vi "Drive Controller.vi"(8 "error in":errorcluster) -> ()   [LabVIEW 2023]
doc: "This VI executes continuously carrying out the current operation and responding to updates or new operation requests. It will often contain the timing or control code that is difficult to place directly in TeleOp. This VI generally opens all sensors and motors and isolates the rest of the robot code from knowing implementation details of how the operations are carried out."
uses:
  Drive Operations.ctl
  bordeaux-pathinator/Bordeaux/Types/Segment Type.ctl
  bordeaux-pathinator/Bordeaux/Types/Limits.ctl
  Drive Setpoints.ctl
  swerve/Type Definitions/Data/Robot Velocities.ctl
  <vilib>/Rock Robotics/WPI/ThirdParty/REV Robotics/REVLib/Typedef/Spark MAX Control Type.ctl
  <vilib>/Rock Robotics/WPI/DriverStation/WPI_DriverStationRobotMode2.ctl
  e7fadf63-5109-474c-80f5-604bef1b4eb3.vi
  80b923c8-6b82-42f9-a8cd-acddf0fa8107.vi
  Framework/Robot Global Data.vi
  <vilib>/Rock Robotics/WPI/ThirdParty/Phoenix-LabVIEW/Pigeon IMU/CTRE_PigeonIMU_GetYPR.vi
  <vilib>/Rock Robotics/Network Tables/NT Write Numeric Array.vi
  <vilib>/Rock Robotics/Network Tables/NT Write String.vi
  <vilib>/Rock Robotics/Network Tables/NT Read Numeric Array.vi
  <vilib>/Rock Robotics/Network Tables/NT Read Number.vi
  <vilib>/Platform/TimedLoop/XDataNode/XDataNode.xnode
  <vilib>/Platform/TimedLoop/XDataNode/nitl_modes.ctl
  <vilib>/Platform/TimedLoop/XDataNode/XDNodeRunTimeDep.lvlib
  <vilib>/Platform/TimedLoop/XDataNode/wakeup.ctl
  <vilib>/Platform/TimedLoop/XDataNode/timing_clust.ctl
  <vilib>/ptbypt/NI_PtbyPt.lvlib
panel:
  out "Error":T1
  in  "Limits":T2={"Velocity (fps)"=10.0, "Accel (fps^2)"=22.0, "Jerk (fps^3)"=4000.0, "StoopidFast (fps)"=10.0} {"StoopidFast (fps)" min=0.0; "Jerk (fps^3)" min=0.0 step=1.0; "Accel (fps^2)" min=0.0; "Velocity (fps)" min=0.0}
  in  "Final Postion":T1={"X setpoint"=13.0, "Y setpoint"=8.0, "Theta"=0.0}
  out "Yaw":dbl=3.92486572265625
  in  "Y Setpoint":dbl=-0.8
  in  "Right PID Setpoint":dbl=0.56
  in  "Left PID Setpoint":dbl=-0.545
  in  "Freeze Align?":bool
  out "VMag Sum":dbl=1.7248000000000006
  out "Enabled VMag":dbl[](graph)=[0.44, 0.88, 1.32, 1.76, 2.2, 2.64, 3.08, 3.52, 3.96, 4.4, 4.840000000000001, 5.280000000000001, 5.7200000000000015, 6.160000000000002, 5.7200000000000015, 5.280000000000001, 4.840000000000001, 4.4, 3.9600000000000004, 3.5200000000000005, 3.0800000000000005, 2.6400000000000006, 2.2000000000000006, 1.7600000000000007, 1.3200000000000007, 1.3200000000000007]
  out "Sum Angle":dbl=-0.25517736196517943
  out "Sum Y":dbl=1.7237185415021776
  out "Sum X":dbl=-0.061040277189923345
  out "Enabled Omega":dbl[](graph)=[-0.0, -0.554733395576477, -0.554733395576477, -0.554733395576477, -0.554733395576477, -0.554733395576477, -0.554733395576477, -0.554733395576477, -0.554733395576477, -0.554733395576477, -0.554733395576477, -0.554733395576477, -0.554733395576477, -0.554733395576477, -0.554733395576477, -0.554733395576477, -0.554733395576477, -0.554733395576477, -0.554733395576477, -0.554733395576477, -0.554733395576477, -0.554733395576477, -0.554733395576477, -0.554733395576477, -0.0, -0.0]
  out "Enabled Y Velocity":dbl[](graph)=[0.4397620571088689, 0.8795184944701074, 1.3192692626162588, 1.7590143120802895, 2.1987535933955944, 2.6384870570959973, 3.0782146537157553, 3.517936333789562, 3.9576520478525503, 4.397361746440296, 4.837065380088821, 5.276762899334593, 5.7164542547145345, 6.1561393967660205, 5.7163758392233, 5.2766181322765675, 4.836866325390256, 4.397120468028349, 3.9573806096543764, 3.5176467997314127, 3.0779190877220737, 2.638197523088511, 2.1984821552924134, 1.7587730337949996, 1.31907977534625, 1.319075836091112]
  out "Enabled X Velocity":dbl[](graph)=[-0.014468349158626874, -0.02910700749021977, -0.04391597335768957, -0.05889524511117701, -0.07404482108804894, -0.0893646996129026, -0.10485487899756332, -0.12051535754108665, -0.13634613352975256, -0.15234720523707615, -0.16851857092379446, -0.1848602288378793, -0.2013721772145311, -0.21805441427617603, -0.2035860131348127, -0.18894731046023522, -0.17413830797893487, -0.1591590074301729, -0.14400941056597527, -0.12868951915114632, -0.1131993349632539, -0.09753885979264178, -0.08170809544241993, -0.06570704372847282, -0.049280282796354616, -0.04938561167522259]
  out "Trajectory Velocity":dbl[](graph)
  out "Trajectory Data Compare":T4(array[cluster])
  out "Trajectory Data Out":T4(array[cluster])=[{"Segment Name"="Linear 0", "Type"=enum."Accel Straight", "Traj Pos Points"=[{"x"=-0.40649778342800347, "y"=-2.496126393436387, "th"=0.25975245237350464}, {"x"=-0.4068270208391716, "y"=-2.4873325545291127, "th"=0.2486577844619751}, {"x"=-0.4074854956615079, "y"=-2.4697448767145644, "th"=0.23756311655044554}, {"x"=-0.40847320789501235, "y"=-2.443363359992742, "th"=0.22646844863891602}, {"x"=-0.40979015753968495, "y"=-2.408188004363646, "th"=0.21537378072738647}, {"x"=-0.4114363445955257, "y"=-2.3642188098272756, "th"=0.20427911281585692}, {"x"=-0.4134117690625346, "y"=-2.311455776383631, "th"=0.1931844449043274}, {"x"=-0.41571643094071165, "y"=-2.2498989040327126, "th"=0.18208977699279785}, {"x"=-0.41835033023005685, "y"=-2.17954819277452, "th"=0.1709951090812683}, {"x"=-0.4213134669305702, "y"=-2.100403642609053, "th"=0.15990044116973876}, {"x"=-0.4246058410422517, "y"=-2.0124652535363126, "th"=0.1488057732582092}, {"x"=-0.42822745256510136, "y"=-1.9157330255562977, "th"=0.13771110534667966}, {"x"=-0.4321783014991192, "y"=-1.8102069586690088, "th"=0.1266164374351501}, {"x"=-0.43645838784430513, "y"=-1.6958870528744459, "th"=0.11552176952362056}, {"x"=-0.4410677116006592, "y"=-1.5727733081726087, "th"=0.10442710161209101}, {"x"=-0.44534779794584517, "y"=-1.4584534023780458, "th"=0.09333243370056146}, {"x"=-0.449298646879863, "y"=-1.352927335490757, "th"=0.08223776578903191}, {"x"=-0.45292025840271266, "y"=-1.256195107510742, "th"=0.07114309787750236}, {"x"=-0.45621263251439415, "y"=-1.1682567184380013, "th"=0.060048429965972816}, {"x"=-0.4591757692149075, "y"=-1.0891121682725347, "th"=0.04895376205444327}, {"x"=-0.4618096685042527, "y"=-1.018761457014342, "th"=0.03785909414291372}, {"x"=-0.4641143303824298, "y"=-0.9572045846634234, "th"=0.02676442623138417}, {"x"=-0.46608975484943865, "y"=-0.904441551219779, "th"=0.01566975831985462}, {"x"=-0.4677359419052794, "y"=-0.8604723566834086, "th"=0.0045750904083251}, {"x"=-0.469052891549952, "y"=-0.8252970010543123, "th"=0.0045750904083251}, {"x"=-0.47004060378345647, "y"=-0.79891548433249, "th"=0.0}], "Traj Vel Points"=[{"V"=0.44, "Omega"=-0.0, "V vector"={"y"=-0.4397620571088689, "x"=-0.014468349158626874}}, {"V"=0.88, "Omega"=-0.554733395576477, "V vector"={"y"=-0.8795184944701074, "x"=-0.02910700749021977}}, {"V"=1.32, "Omega"=-0.554733395576477, "V vector"={"y"=-1.3192692626162588, "x"=-0.04391597335768957}}, {"V"=1.76, "Omega"=-0.554733395576477, "V vector"={"y"=-1.7590143120802895, "x"=-0.05889524511117701}}, {"V"=2.2, "Omega"=-0.554733395576477, "V vector"={"y"=-2.1987535933955944, "x"=-0.07404482108804894}}, {"V"=2.64, "Omega"=-0.554733395576477, "V vector"={"y"=-2.6384870570959973, "x"=-0.0893646996129026}}, {"V"=3.08, "Omega"=-0.554733395576477, "V vector"={"y"=-3.0782146537157553, "x"=-0.10485487899756332}}, {"V"=3.52, "Omega"=-0.554733395576477, "V vector"={"y"=-3.517936333789562, "x"=-0.12051535754108665}}, {"V"=3.96, "Omega"=-0.554733395576477, "V vector"={"y"=-3.9576520478525503, "x"=-0.13634613352975256}}, {"V"=4.4, "Omega"=-0.554733395576477, "V vector"={"y"=-4.397361746440296, "x"=-0.15234720523707615}}, {"V"=4.840000000000001, "Omega"=-0.554733395576477, "V vector"={"y"=-4.837065380088821, "x"=-0.16851857092379446}}, {"V"=5.280000000000001, "Omega"=-0.554733395576477, "V vector"={"y"=-5.276762899334593, "x"=-0.1848602288378793}}, {"V"=5.7200000000000015, "Omega"=-0.554733395576477, "V vector"={"y"=-5.7164542547145345, "x"=-0.2013721772145311}}, {"V"=6.160000000000002, "Omega"=-0.554733395576477, "V vector"={"y"=-6.1561393967660205, "x"=-0.21805441427617603}}, {"V"=5.7200000000000015, "Omega"=-0.554733395576477, "V vector"={"y"=-5.7163758392233, "x"=-0.2035860131348127}}, {"V"=5.280000000000001, "Omega"=-0.554733395576477, "V vector"={"y"=-5.2766181322765675, "x"=-0.18894731046023522}}, {"V"=4.840000000000001, "Omega"=-0.554733395576477, "V vector"={"y"=-4.836866325390256, "x"=-0.17413830797893487}}, {"V"=4.4, "Omega"=-0.554733395576477, "V vector"={"y"=-4.397120468028349, "x"=-0.1591590074301729}}, {"V"=3.9600000000000004, "Omega"=-0.554733395576477, "V vector"={"y"=-3.9573806096543764, "x"=-0.14400941056597527}}, {"V"=3.5200000000000005, "Omega"=-0.554733395576477, "V vector"={"y"=-3.5176467997314127, "x"=-0.12868951915114632}}, {"V"=3.0800000000000005, "Omega"=-0.554733395576477, "V vector"={"y"=-3.0779190877220737, "x"=-0.1131993349632539}}, {"V"=2.6400000000000006, "Omega"=-0.554733395576477, "V vector"={"y"=-2.638197523088511, "x"=-0.09753885979264178}}, {"V"=2.2000000000000006, "Omega"=-0.554733395576477, "V vector"={"y"=-2.1984821552924134, "x"=-0.08170809544241993}}, {"V"=1.7600000000000007, "Omega"=-0.554733395576477, "V vector"={"y"=-1.7587730337949996, "x"=-0.06570704372847282}}, {"V"=1.3200000000000007, "Omega"=-0.0, "V vector"={"y"=-1.31907977534625, "x"=-0.049280282796354616}}, {"V"=1.3200000000000007, "Omega"=-0.0, "V vector"={"y"=-1.319075836091112, "x"=-0.04938561167522259}}], "Accel Index"=14, "Decel Index"=14}, {"Segment Name"="", "Type"=enum."Accel Straight", "Traj Pos Points"=[], "Traj Vel Points"=[], "Accel Index"=0, "Decel Index"=0}]
  in  "PID enabled":bool=TRUE
  out "Trapezoid Profile":dbl[](graph)
  out "Weird Aligning Code?":string
  in  "Go Up?":i32
  in  "Int per ft":dbl=0.75
  in  "PID gains":T5={"proportional gain (Kp)"=1.5, "integral time (Ki)"=0.075, "derivative time (Kd)"=0.0} {"derivative time (Kd)" format="%.3f"; "integral time (Ki)" format="%.3f"; "proportional gain (Kp)" format="%.3f"}
  out "PID Out":dbl=0.10498956284304024
  out "Waveform Chart":cluster{dbl, "Right X Setpoint":dbl}(graph)={-0.574331443611901, "Right X Setpoint"=-0.559167}
  in  "Operation":T6
  in  "Auto PID Constants":T7={"P Gain"=0.09, "I Gain"=0.0, "D Gain"=0.0, "F Gain"=0.08, "I Zone"=0.0, "Min Output"=-1.0, "Max Output"=1.0}
  in  "Immediate PID Constants":T7={"P Gain"=0.09, "I Gain"=0.0, "D Gain"=0.0, "F Gain"=0.08, "I Zone"=0.0, "Min Output"=-1.0, "Max Output"=1.0}
  out "Waveform Chart":cluster{"Numeric":dbl, "Numeric":dbl}(graph)
  in  "Period":i32=26
  in  "Acceleration Max":dbl=3.0
  in  "Velocity Max":dbl=6.0
  in  "Left X Setpoint":dbl=-0.47
  in  "Left Y Setpoint":dbl
  in  "Right Y Setpoint":dbl
  in  "Right X Setpoint":dbl=0.47
  in  "Deadband":T8={"Angle (deg)"=3.0, "X (ft)"=0.1, "Y (ft)"=0.125}
  in  "Drive Controller Diagnostics":T9(tab)
  out "Swerve Visualizer":cluster{dbl[], dbl[]}[](graph)
  out "Pod Comparisons (Diff -> Setpoint - Actual)":T10
  out "(Calibration) Steering Angles":T11={"Left Front"=97.29912567138672, "Left Back"=4.939062595367432, "Right Front"=-174.1834259033203, "Right Back"=-81.83795166015625}
  out "Current\nCmd":string="Started at  16:32:32.148\n: Immediate,  Vx 0.0, Vy -0.0, W -0.000000"
  # "Align Variables"
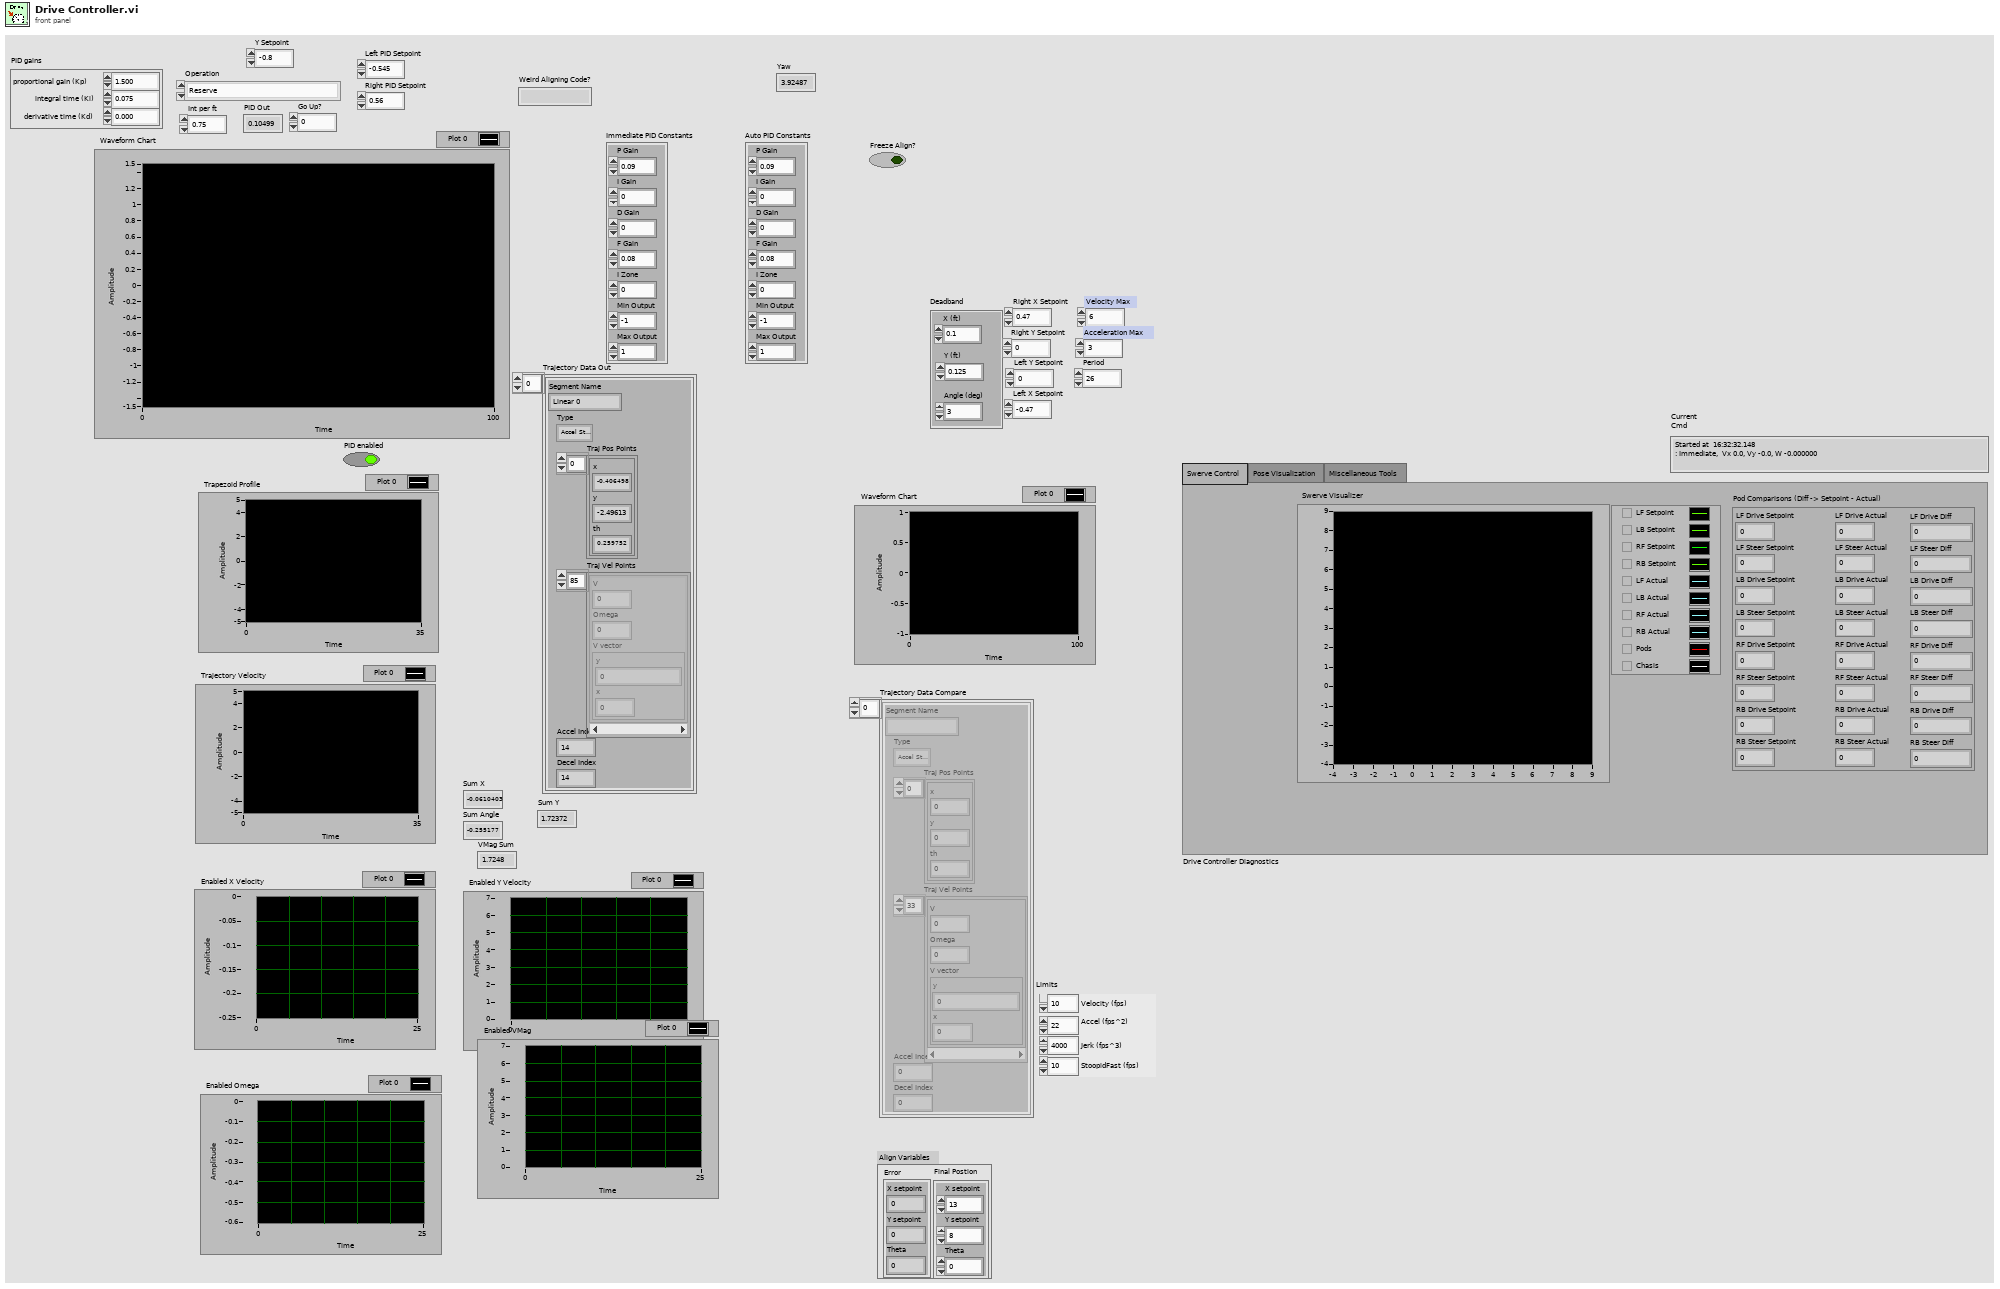
[diagram p1: front panel]
types:
  T1 = cluster{"X setpoint":dbl, "Y setpoint":dbl, "Theta":dbl}
  T2 = typedef "Limits.ctl" = cluster{"Velocity (fps)":dbl, "Accel (fps^2)":dbl, "Jerk (fps^3)":dbl, "StoopidFast (fps)":dbl}
  T3 = typedef "Segment Type.ctl" = enum16{"Accel Straight", "Const Straight", "Blend", "Circle", "Bezier"}
  T4 = cluster{"Segment Name":string, "Type":T3, "Traj Pos Points":cluster{"x":dbl, "y":dbl, "th":dbl}[], "Traj Vel Points":cluster{"V":dbl, "Omega":dbl, "V vector":cluster{"y":dbl, "x":dbl}}[], "Accel Index":i32, "Decel Index":i32}[]
  T5 = cluster{"proportional gain (Kp)":dbl, "integral time (Ki)":dbl, "derivative time (Kd)":dbl}
  T6 = typedef "Drive Operations.ctl" = enum16{"Reserve", "Read Current", "Immediate", "Calibrate", "Reef Align", "Auto", "Old Reef Align"}
  T7 = cluster{"P Gain":dbl, "I Gain":dbl, "D Gain":dbl, "F Gain":dbl, "I Zone":dbl, "Min Output":dbl, "Max Output":dbl}
  T8 = cluster{"Angle (deg)":dbl, "X (ft)":dbl, "Y (ft)":dbl}
  T9 = enum32{"Swerve Control", "Pose Visualization", "Miscellaneous Tools"}
  T10 = cluster{"LF Drive Setpoint":dbl, "LF Steer Setpoint":dbl, "LB Drive Setpoint":dbl, "LB Steer Setpoint":dbl, "RF Drive Setpoint":dbl, "RF Steer Setpoint":dbl, "RB Drive Setpoint":dbl, "RB Steer Setpoint":dbl, "LF Drive Actual":dbl, "LF Steer Actual":dbl, "LB Drive Actual":dbl, "LB Steer Actual":dbl, "RF Drive Actual":dbl, "RF Steer Actual":dbl, "RB Drive Actual":dbl, "RB Steer Actual":dbl, "LF Drive Diff":dbl, "LF Steer Diff":dbl, "LB Drive Diff":dbl, "LB Steer Diff":dbl, "RF Drive Diff":dbl, "RF Steer Diff":dbl, "RB Drive Diff":dbl, "RB Steer Diff":dbl}
  T11 = cluster{"Left Front":dbl, "Left Back":dbl, "Right Front":dbl, "Right Back":dbl}
  T12 = typedef "Drive Setpoints.ctl" = cluster{"Operation":T6, "Robot Velocities":T13, "Auto Data":cluster{"Auto Velocities":T13[], "Auto Positions":cluster{"x":dbl, "y":dbl, "th":dbl}[], "Auto Commands":cluster{dbl, "Command out":cluster{"Name":string, "vi reference":refnum<vi>, i32[], variant[]}}[], "Zero Velocity?":bool[]}, "Left side":bool, "Angle Align":bool, "Tag ID":i32}
  T13 = typedef "Robot Velocities.ctl" = cluster{"X Velocity":dbl, "Y Velocity":dbl, "Rotational \nVelocity":dbl}
  T14 = typedef "(NEO-NEO-ThroughBore-Pigeon2) Swerve.ctl" = cluster{"Drive Motors (NEO)":T15, "Steer Motors (NEO)":T15, "Pigeon2":T21, "Radii (ft)":T23}
  T15 = typedef "(NEO & NEO 550) 4 Motor Set.ctl" = cluster{"Left Front":T16, "Left Back":T16, "Right Front":T16, "Right Back":T16}
  T16 = typedef "WPI_MotorControlDeviceRef.ctl" = cluster{"DeviceStatus":errorcluster, "Type":T17, "PWM":cluster{"PWM Channel":T18, "DeadBand":T19}, "CAN":cluster{"Device Number":u8, "SetOutput VI Ref":variant, "GetOutput VI Ref":variant, "Enable VI Ref":variant, "Disable VI Ref":variant, "Data":variant}, "Invert":bool, "DIO PWM":cluster{"PWM \"Enable\" Channel":T18, "DIOChannel":T20, "PWM Rate":dbl}}
  T17 = typedef "WPI_MotorControlType.ctl" = enum16{"PWM", "CAN", "DIO PWM"}
  T18 = typedef "FPGA_DIOPWMChannel.ctl" = enum8{"PWM 0", "PWM 1", "PWM 2", "PWM 3", "PWM 4", "PWM 5", "PWM 6", "PWM 7", "PWM 8", "PWM 9", "PWM MXP 0", "PWM MXP 1", "PWM MXP 2", "PWM MXP 3", "PWM MXP 4", "PWM MXP 5", "PWM MXP 6", "PWM MXP 7", "PWM MXP 8", "PWM MXP 9", "Invalid"}
  T19 = typedef "WPI_PWMDeadband.ctl" = cluster{"Name":string, "maxPositivePwm":i32, "minPositivePwm":i32, "centerPwm":i32, "maxNegativePwm":i32, "minNegativePwm":i32, "angularRange":u16}
  T20 = typedef "FPGA_DIOChannel.ctl" = enum8{"DIO 0", "DIO 1", "DIO 2", "DIO 3", "DIO 4", "DIO 5", "DIO 6", "DIO 7", "DIO 8", "DIO 9", "DIO MXP 0", "DIO MXP 1", "DIO MXP 2", "DIO MXP 3", "DIO MXP 4", "DIO MXP 5", "DIO MXP 6", "DIO MXP 7", "DIO MXP 8", "DIO MXP 9", "DIO MXP 10", "DIO MXP 11", "DIO MXP 12", "DIO MXP 13", "DIO MXP 14", "DIO MXP 15", "SPI Port CS1", "SPI Port CS2", "SPI Port CS3", "SPI Port MISO", "SPI Port MOSI", "Invalid"}
  T21 = typedef "CTRE_PigeonIMU_DeviceRef.ctl" = cluster{"DeviceStatus":errorcluster, "Device Number":u8, "Type":T22, "Device ID":u32, "Handle":u64, "UsageFrame":u32, "Library Path":path}
  T22 = typedef "CTRE_PigeonIMU_ConnectionType.ctl" = u32
  T23 = typedef "Pod Positions.ctl" = cluster{"Left Front Position":dbl[], "Left Back Position":dbl[], "Right Front Position":dbl[], "Right Back Position":dbl[]}
  T24 = typedef "Command Status Info.ctl" = cluster{"Name":string, "Status":T25, "notifier out":T26}
  T25 = typedef "Completion Status.ctl" = enum16{"Successful", "Aborted", "Incomplete"}
  T26 = typedef "Completion Notifier.ctl" = refnum<notifier>
  T27 = cluster{"SubSystem Data":T12, cluster{"Start Time (ms)":u32, "Iterations":i32}, cluster{"Command Info":T24, "Description":string, "Default Command":T12, "queue out":refnum<queue>, "Subsystem Name":string}}
  T28 = typedef "Spark MAX Control Type.ctl" = enum16{"Percent VBus", "Voltage", "Velocity", "Position", "Smart Motion", "Current", "Smart Velocity", "MAXMotion Position", "MAXMotion Velocity"}
  T29 = typedef "WPI_DriverStationRobotMode2.ctl" = enum16{"Autonomous Disabled", "Autonomous Enabled", "Teleop Disabled", "Teleop Enabled", "Disconnected", "Finish", "Test Disabled", "Test Enabled", "Emergency Stopped"}
  T30 = typedef "XDNodeRunTimeDep.lvlib/timing_clust.ctl" = cluster{"Expected End [f-1]":u64, "Actual End [f-1]":u64, "Finished Late? [f-1]":bool, "Expected End [i-1]":u64, "Actual End [i-1]":u64, "Finished Late? [i-1]":bool, "Expected Start [i]":u64, "Actual Start [i]":u64, "Expected Start [f]":u64, "Actual Start [f]":u64, "Source Name":string, "Structure Name":string, "Period":i64, "Deadline":i64, "Offset":i64, "Start":i64, "Priority":i32, "Timeout":i32, "Mode":T31, "Wakeup Reason":T32, "Error":errorcluster, "Source Type":string, "Secondary Source Type":string, "Global End Time":u64, "Global Start Time":u64, "Frame Duration":u64, "Iteration Duration":u64, "Assigned CPU":i32, "I/O Scan Engine Mode":u32}
  T31 = typedef "XDNodeRunTimeDep.lvlib/nitl_modes.ctl" = enum32{"No Change", "Process missed periods, maintain original phase", "Discard missed periods, maintain original phase", "Process missed periods, ignore original phase", "Discard missed periods, ignore original phase"}
  T32 = typedef "XDNodeRunTimeDep.lvlib/wakeup.ctl" = enum32{"Normal", "Aborted", "Asynchronous wakeup", "Timing source error", "Timed loop error", "Timeout"}
  T33 = cluster{"Auto Velocities":T13[], "Auto Positions":cluster{"x":dbl, "y":dbl, "th":dbl}[], "Auto Commands":cluster{dbl, "Command out":cluster{"Name":string, "vi reference":refnum<vi>, i32[], variant[]}}[], "Zero Velocity?":bool[]}
  T34 = cluster{"Field Centric":bool, "Reef Centric":bool}
  T35 = typedef "Pod Setpoints.ctl" = cluster{"Left Front":cluster{"Velocity":dbl, "Theta":dbl}, "Left Back":cluster{"Velocity":dbl, "Theta":dbl}, "Right Front":cluster{"Velocity":dbl, "Theta":dbl}, "Right Back":cluster{"Velocity":dbl, "Theta":dbl}}
  T36 = cluster{"Left X Setpoint":dbl, "Left Y Setpoint":dbl}
  T37 = cluster{"Right X Setpoint":dbl, "Right Y Setpoint":dbl}
  T38 = cluster{"Segment Name":string, "Type":T3, "Traj Pos Points":cluster{"x":dbl, "y":dbl, "th":dbl}[], "Traj Vel Points":cluster{"V":dbl, "Omega":dbl, "V vector":cluster{"y":dbl, "x":dbl}}[], "Accel Index":i32, "Decel Index":i32}
  T39 = cluster{"V":dbl, "Omega":dbl, "V vector":cluster{"y":dbl, "x":dbl}}[]
  T40 = cluster{"Filtered x":dbl, "Right X Setpoint":dbl}
  T41 = cluster{"Right X Setpoint":dbl, "Y Setpoint":dbl, dbl}
  T42 = cluster{"x setpoint":dbl, "y setpoint":dbl, "th setpoint":dbl}
  T43 = cluster{"SubSystem Data":T12, cluster{"Start Time (ms)":u32, "Iterations":i32}, "Default Command Arguments":cluster{"Command Info":T24, "Description":string, "Default Command":T12, "queue out":refnum<queue>, "Subsystem Name":string}}
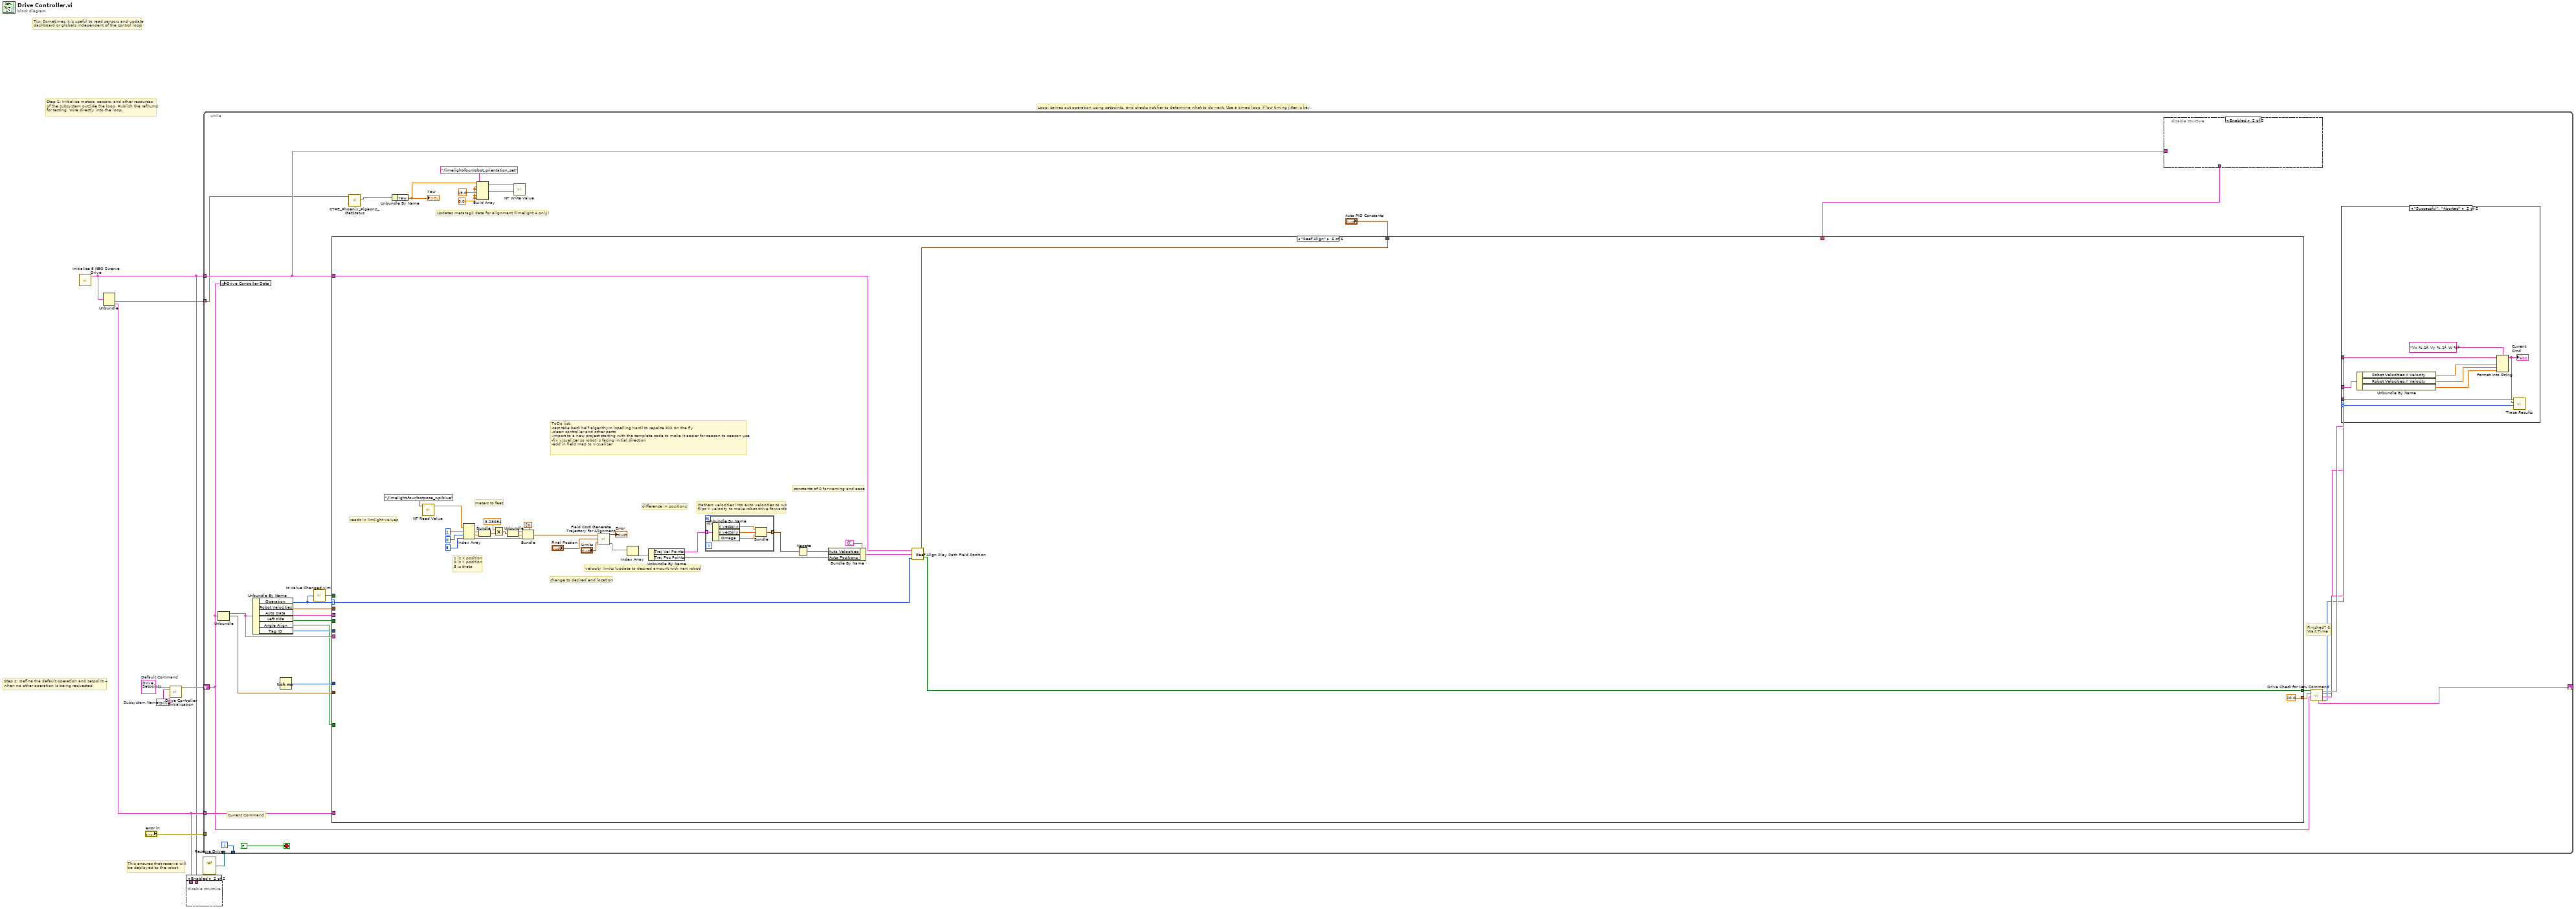
[diagram p0: block diagram]
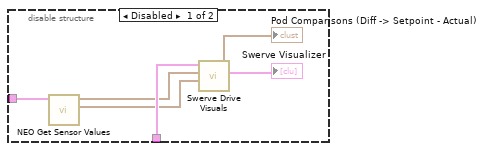
[diagram p2: hidden frame]
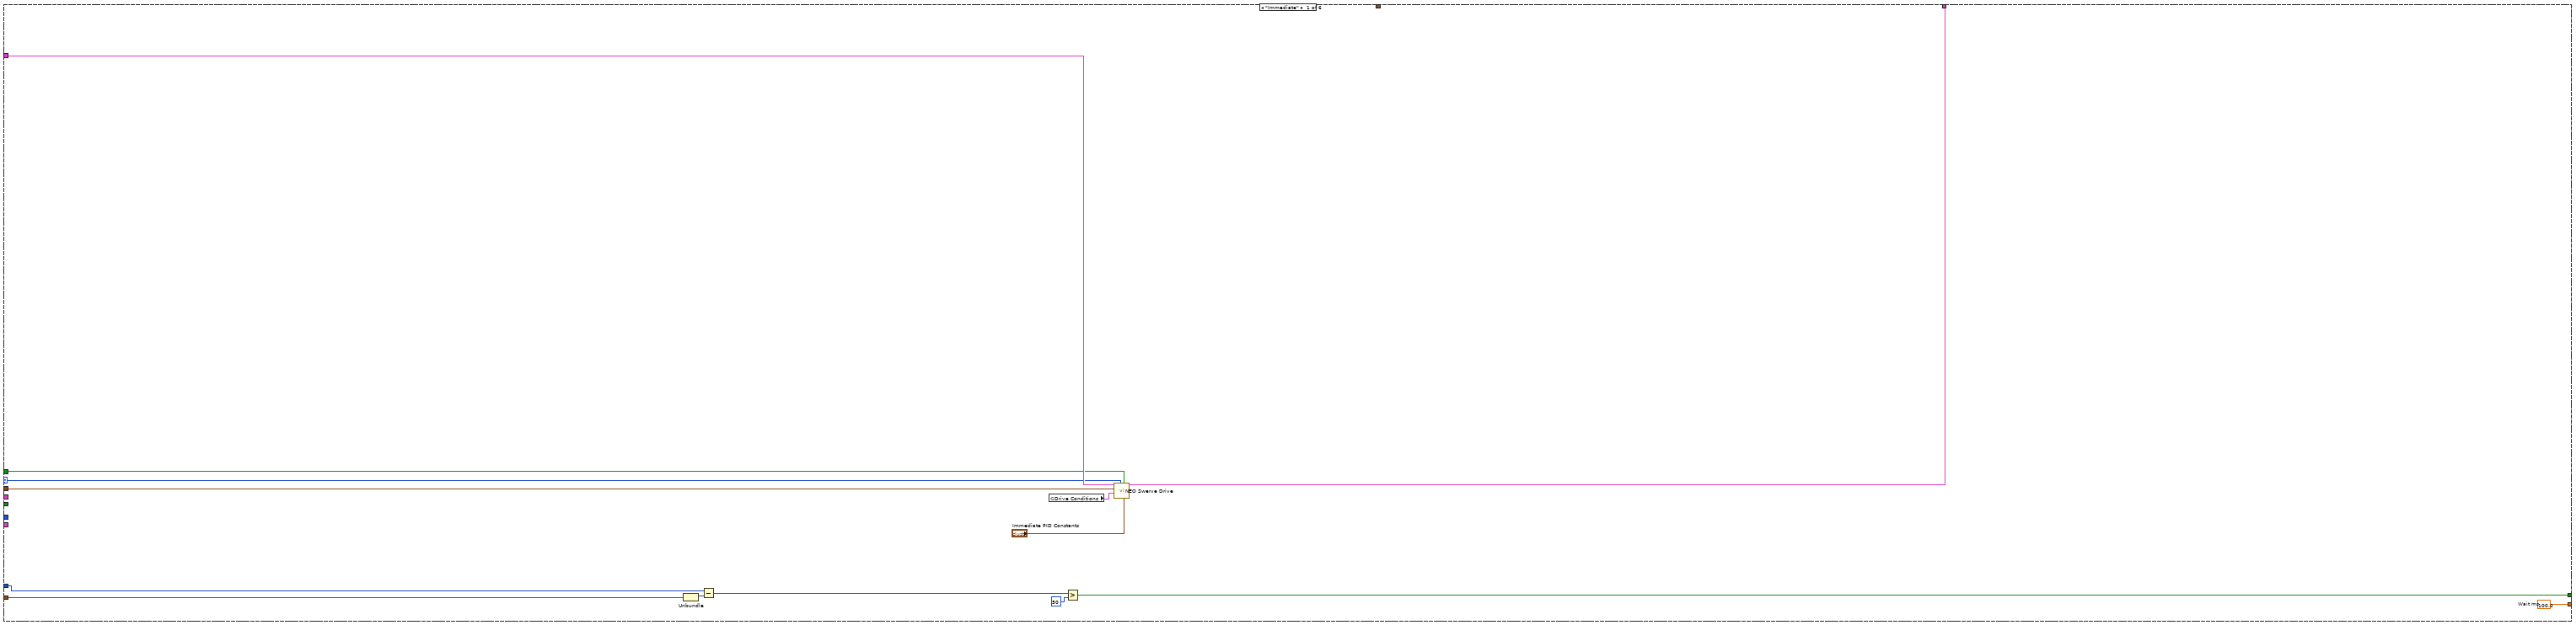
[diagram p3: hidden frame]
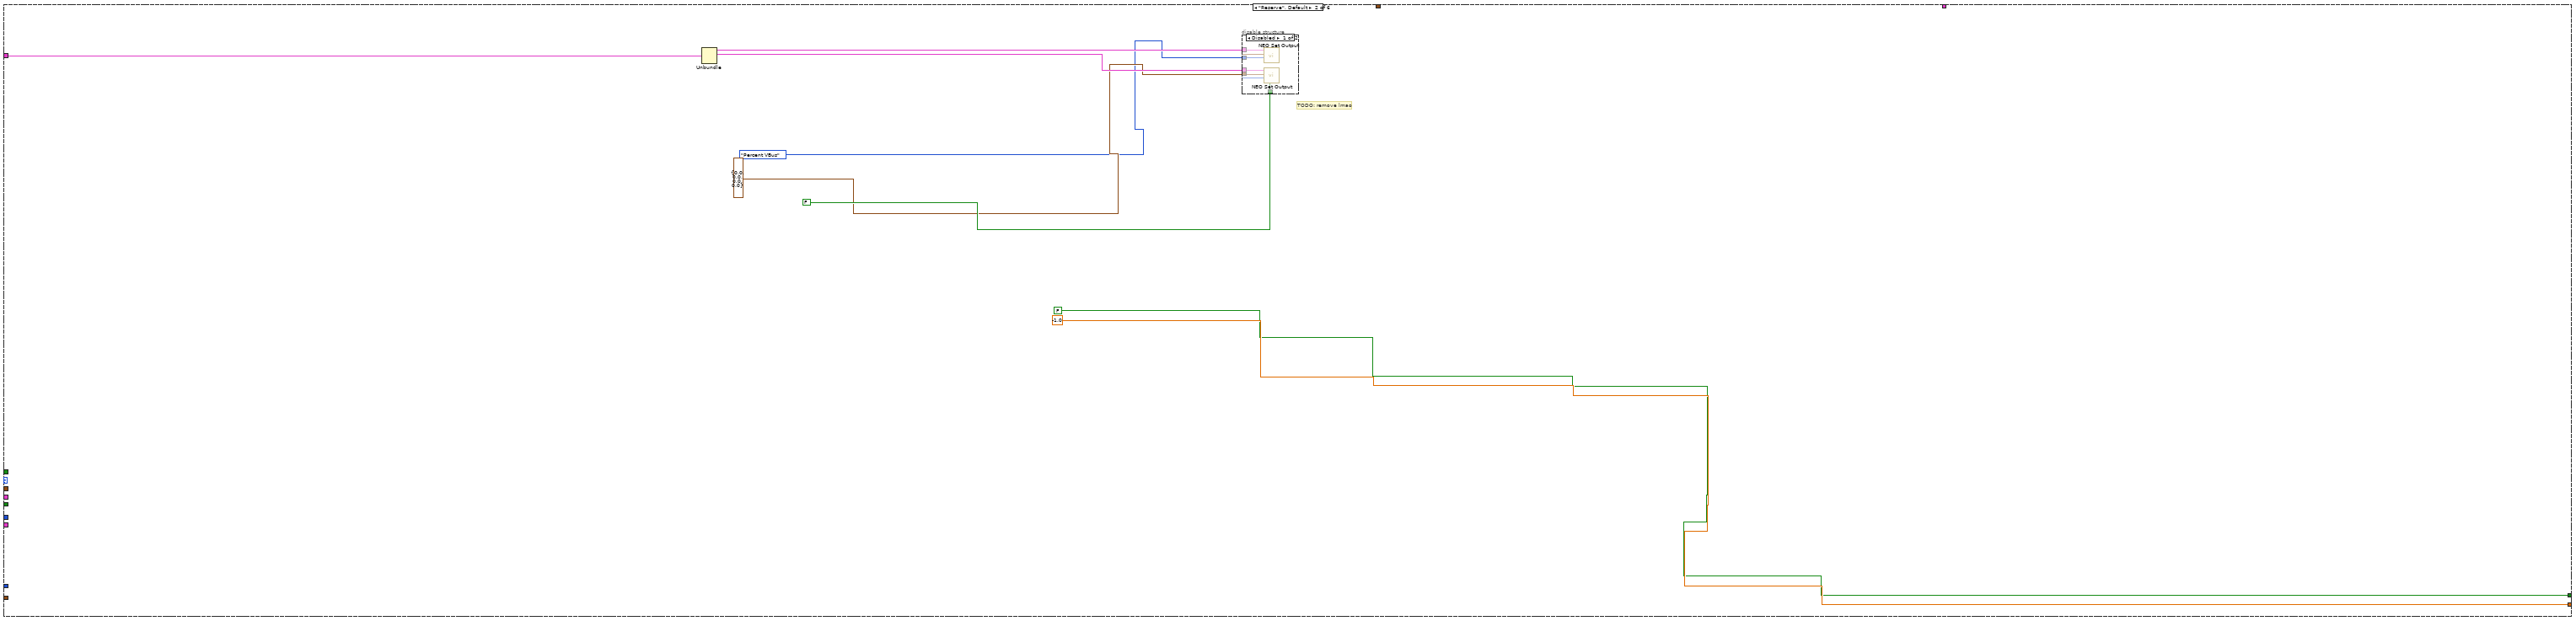
[diagram p4: hidden frame]
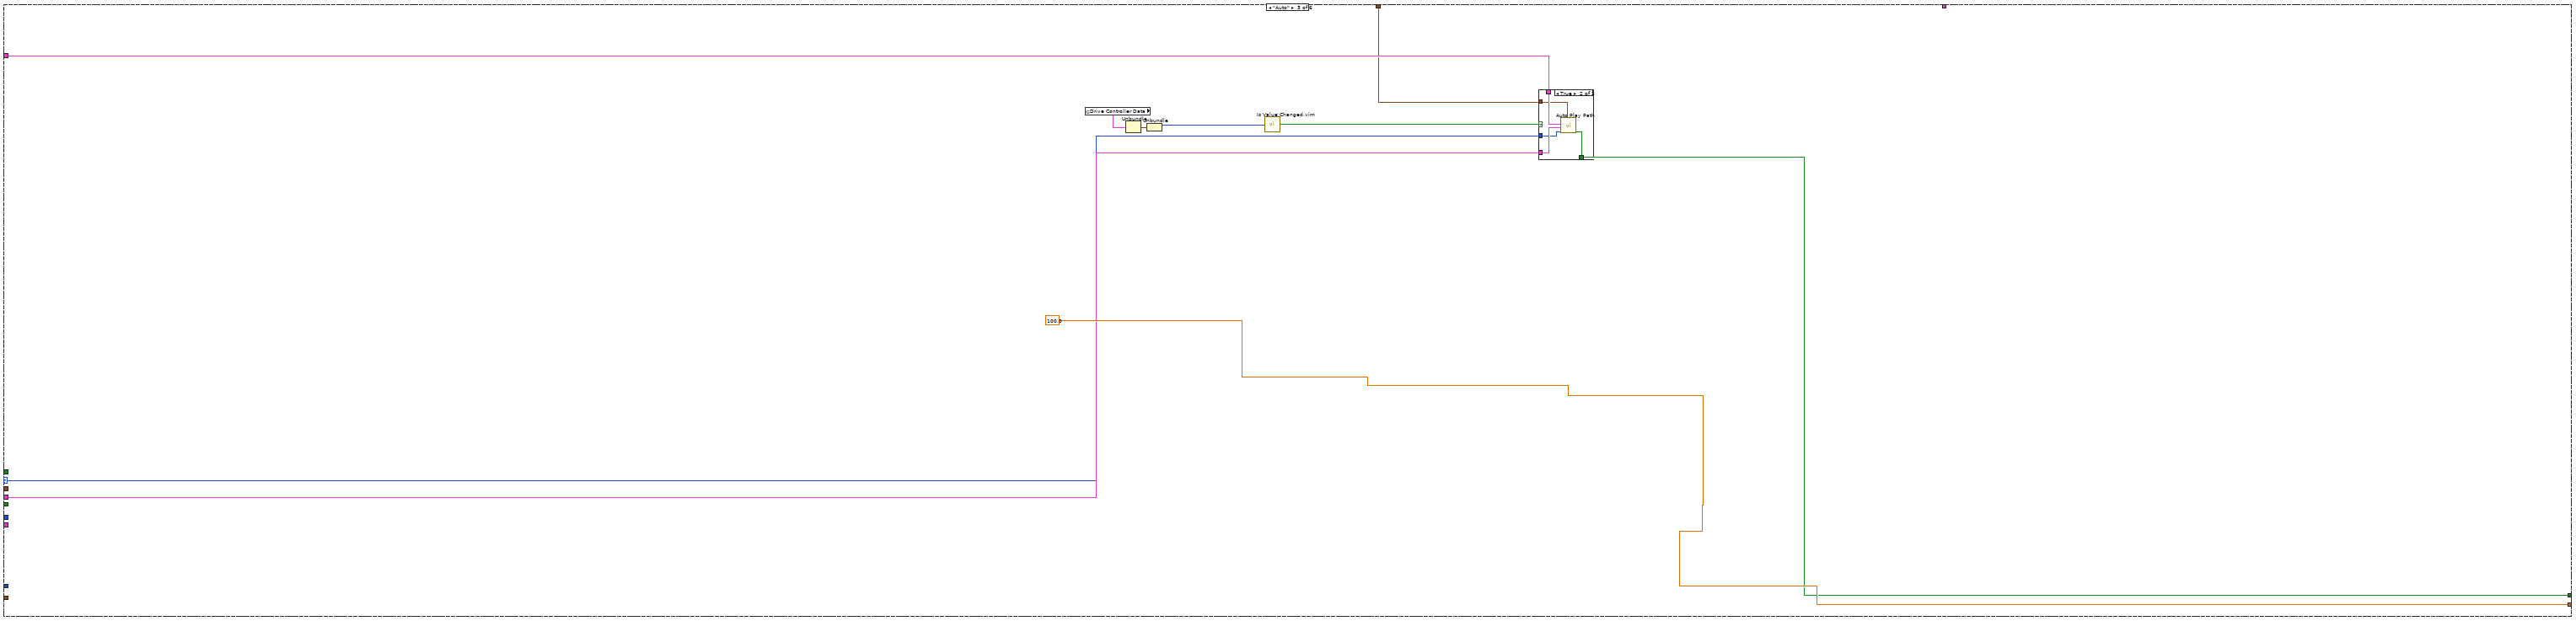
[diagram p6: hidden frame]
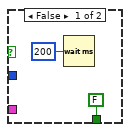
[diagram p7: hidden frame]
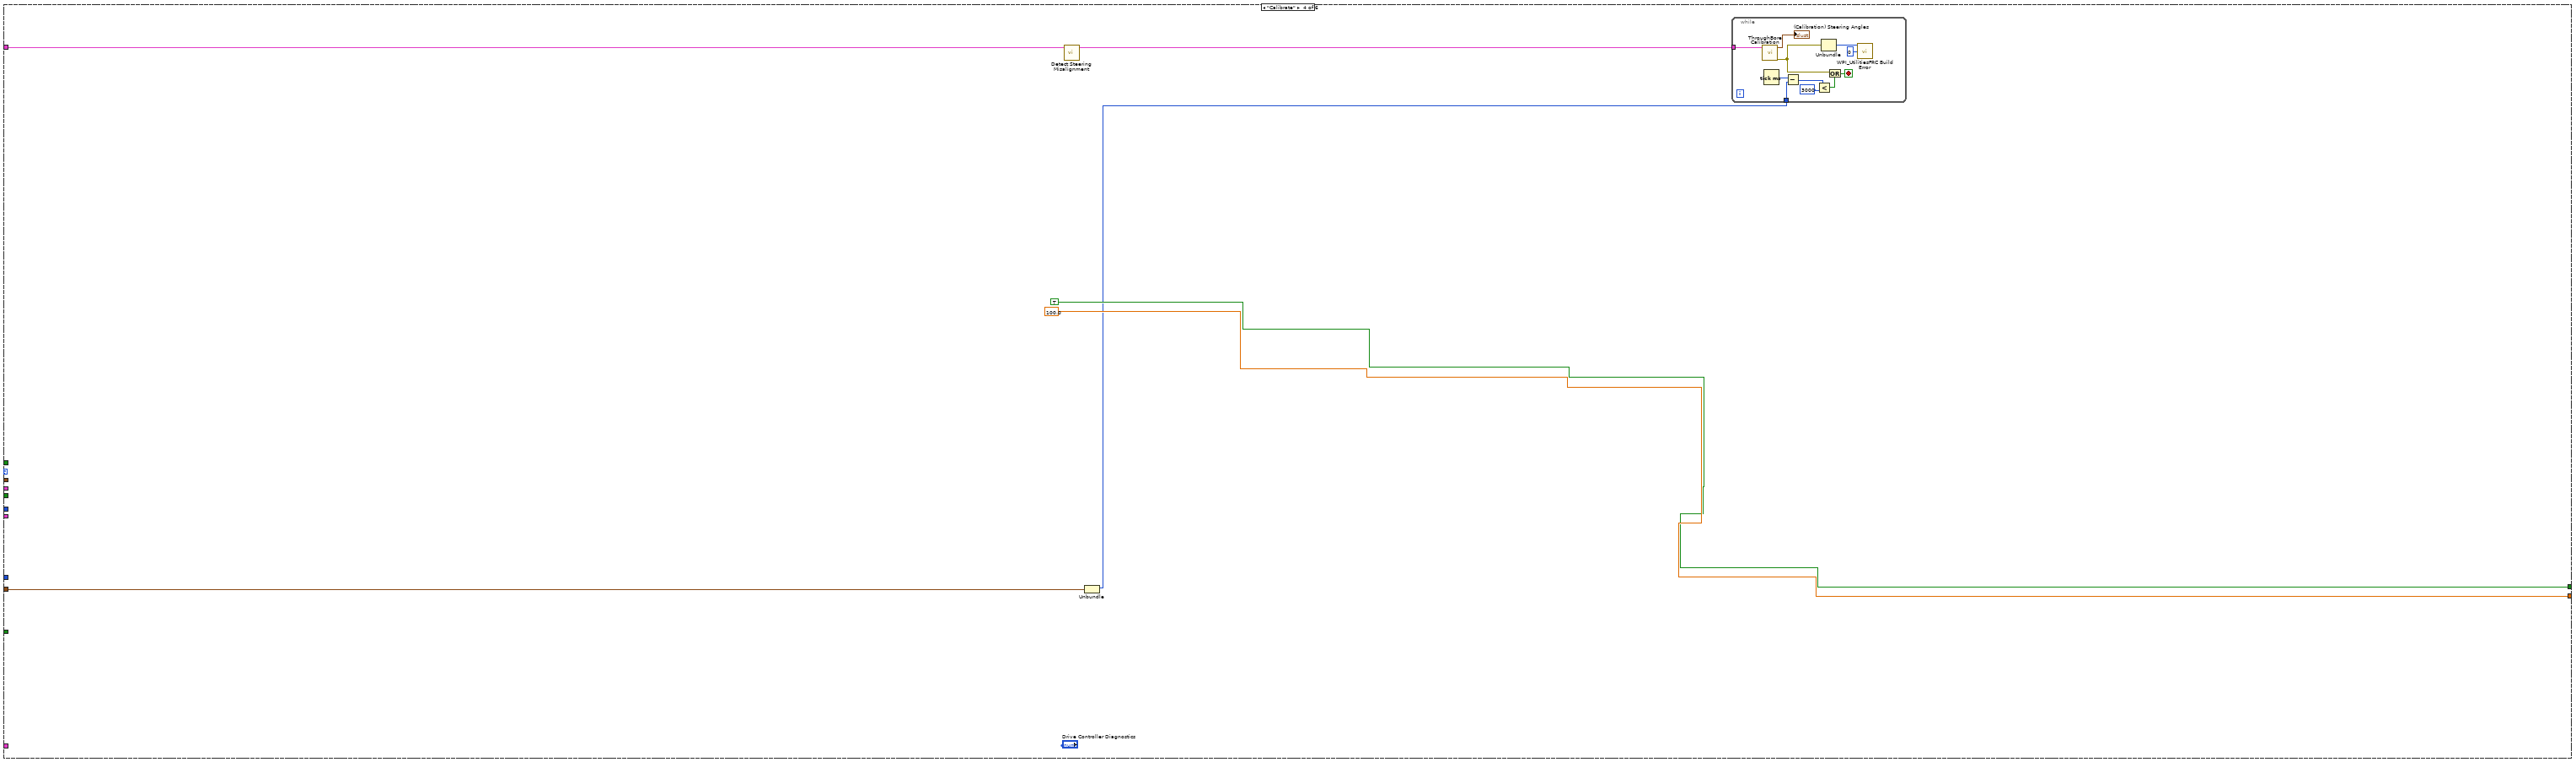
[diagram p8: hidden frame]
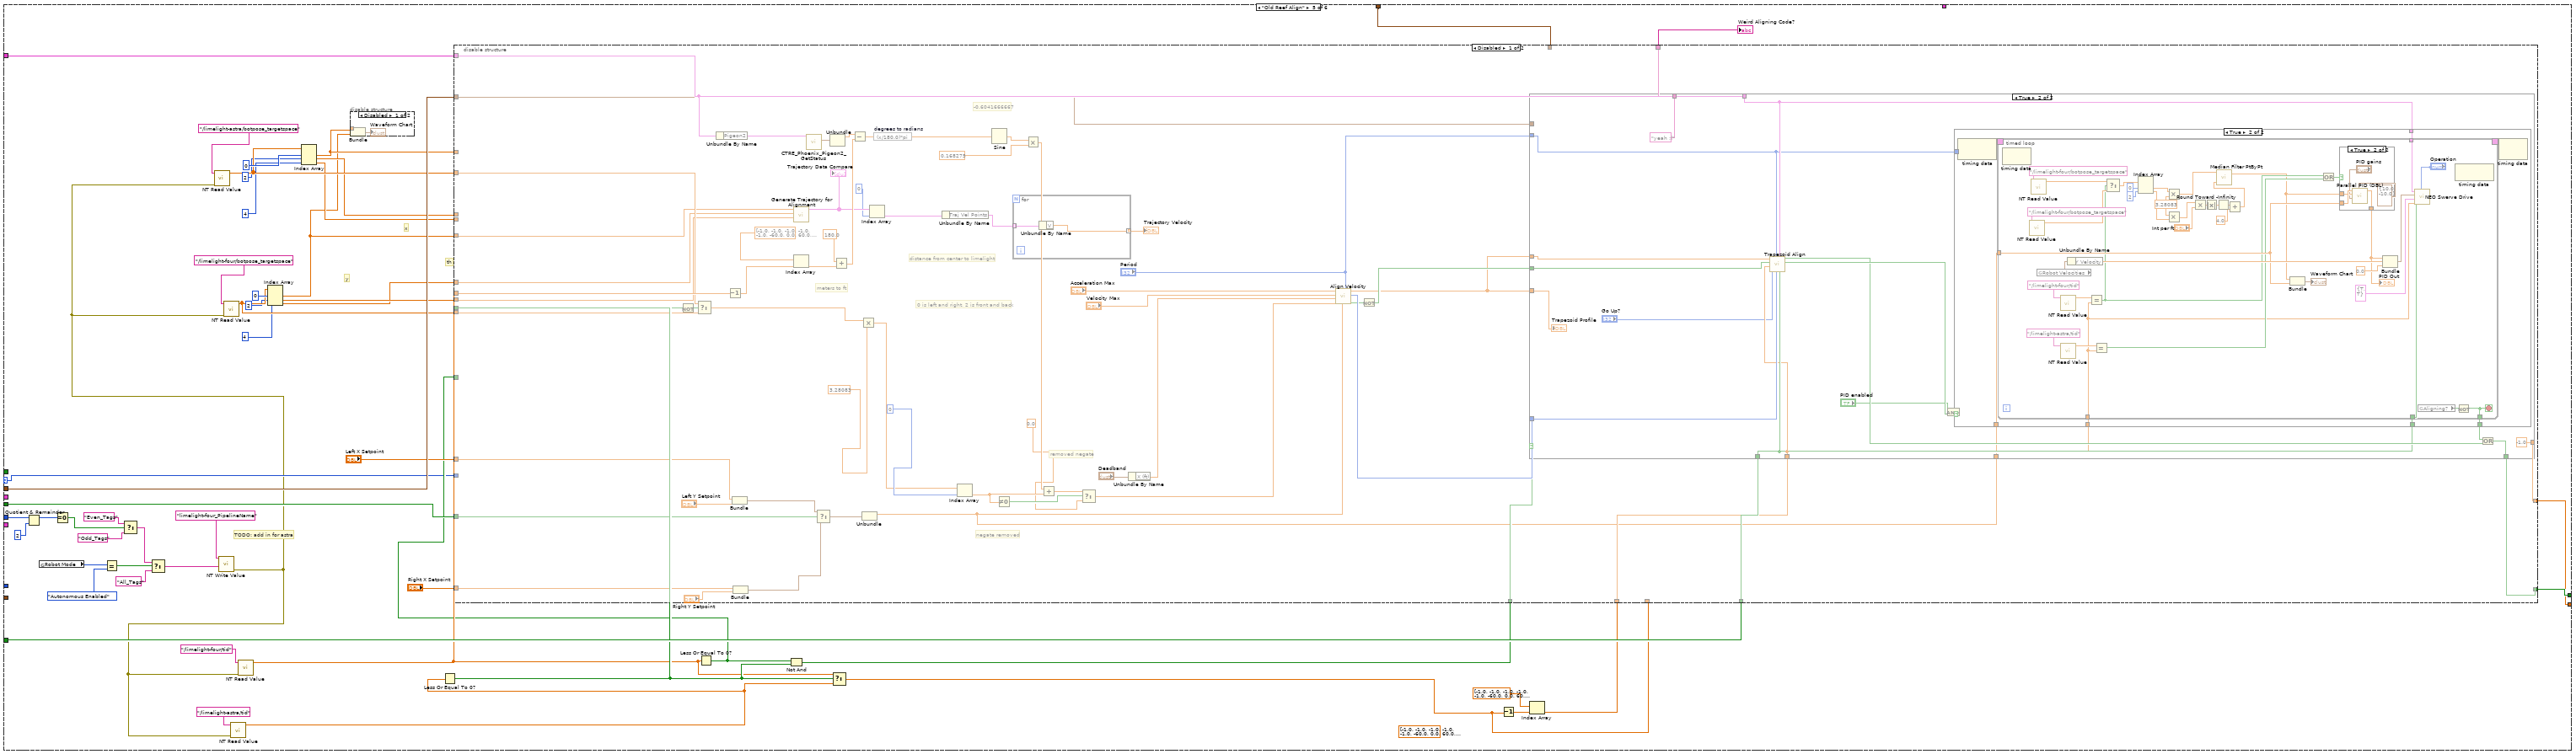
[diagram p9: hidden frame]
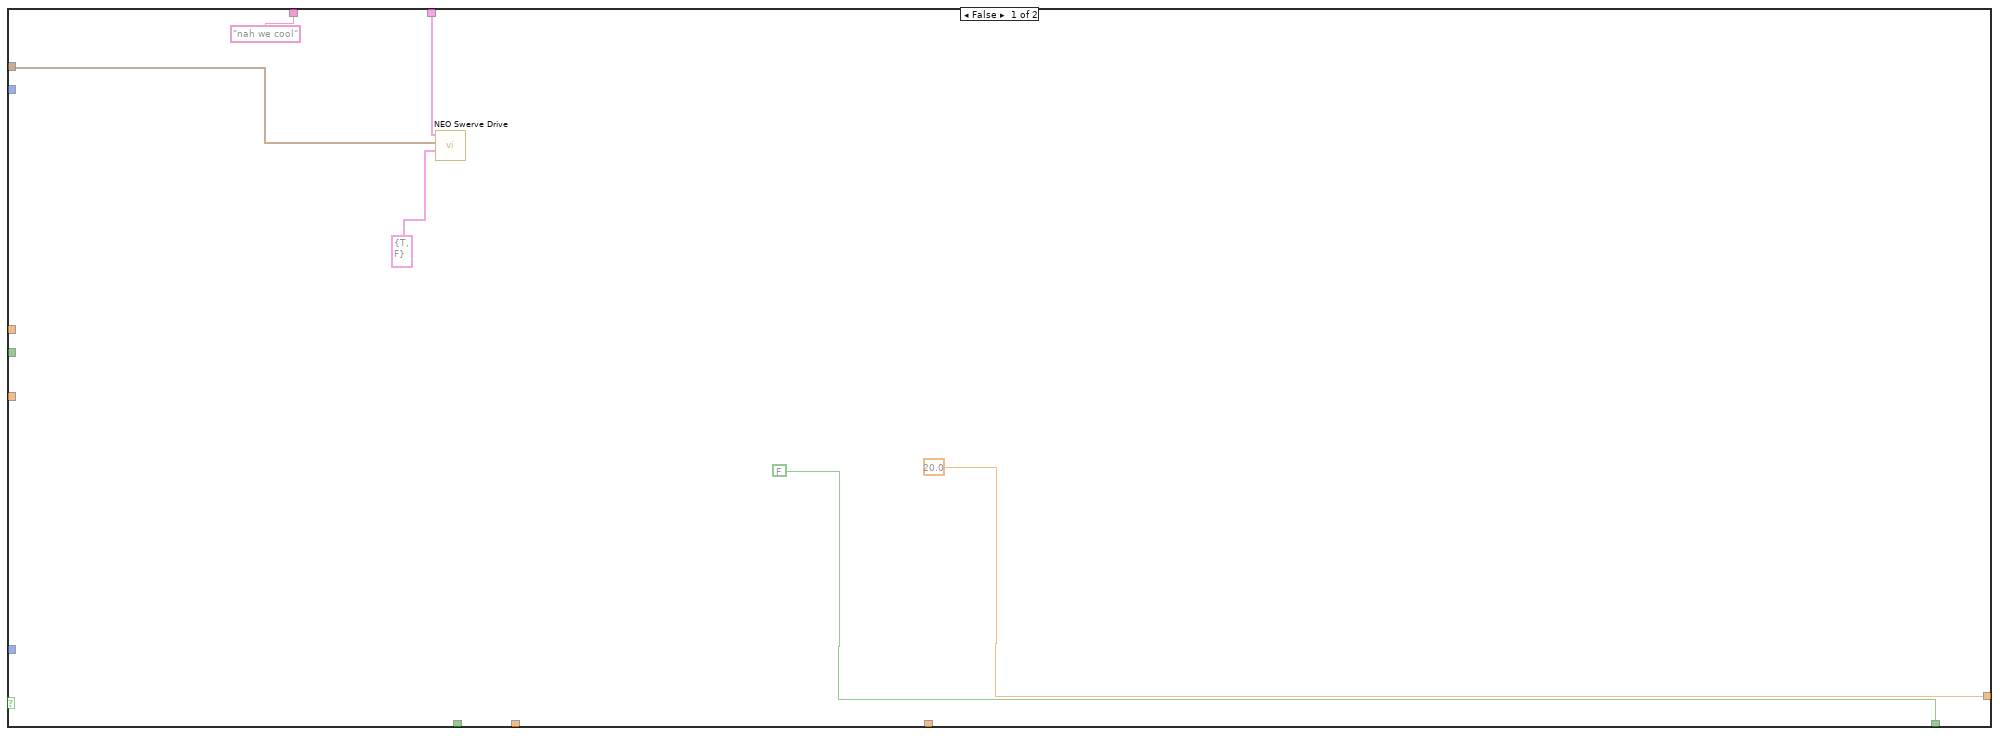
[diagram p11: hidden frame]
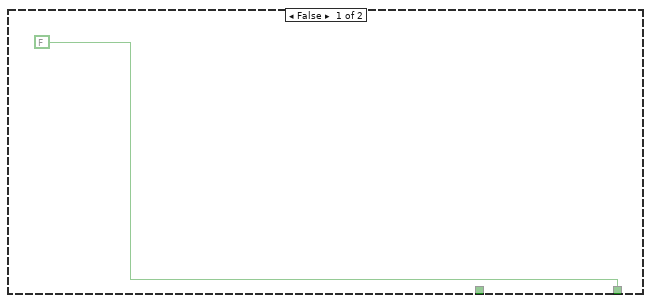
[diagram p12: hidden frame]
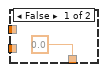
[diagram p13: hidden frame]
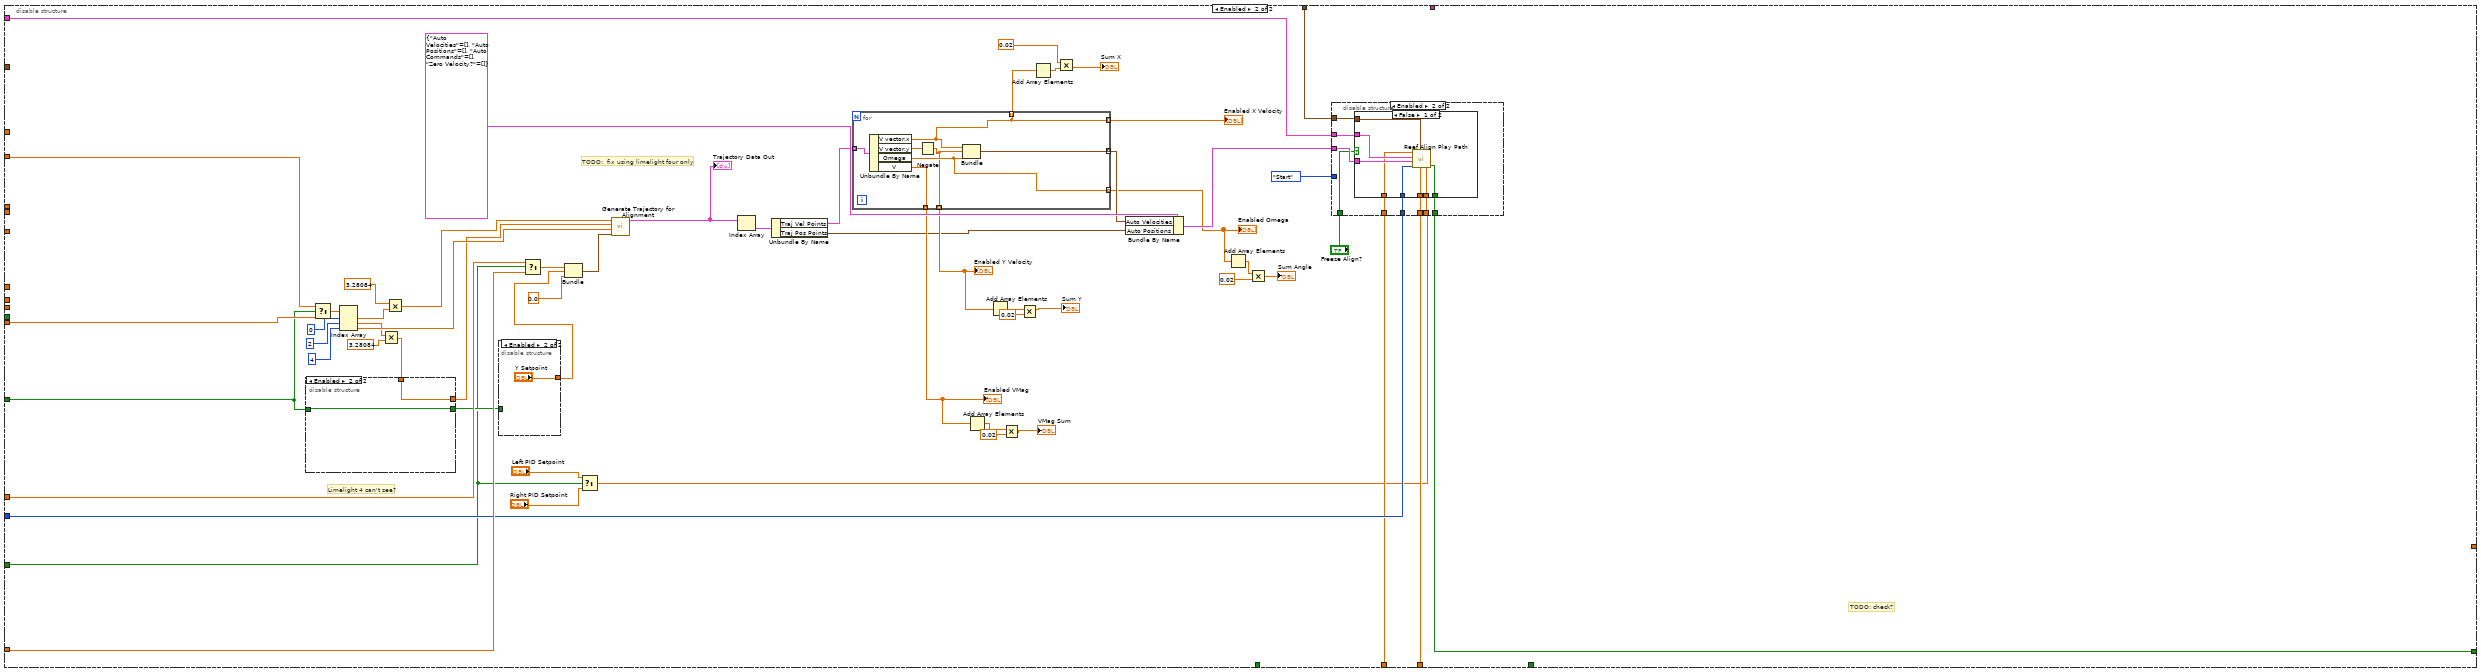
[diagram p14: hidden frame]
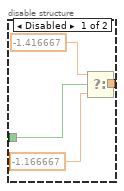
[diagram p15: hidden frame]
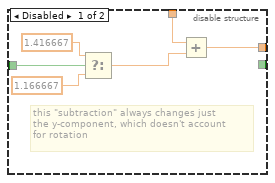
[diagram p16: hidden frame]
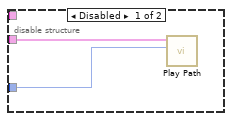
[diagram p17: hidden frame]
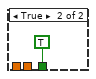
[diagram p18: hidden frame]
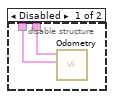
[diagram p20: hidden frame]
diagram:
  w4 = T12 {"Operation"=enum."Reserve", "Robot Velocities"={"X Velocity"=0.0, "Y Velocity"=0.0, "Rotational \nVelocity"=0.0}, "Auto Data"={"Auto Velocities"=[], "Auto Positions"=[], "Auto Commands"=[], "Zero Velocity?"=[]}, "Left side"=FALSE, "Angle Align"=FALSE, "Tag ID"=0}  # Default Command
  w8 = "Drive"  # Subsystem Name
  # "This ensures that reserve will\nbe deployed to the robot"
  # "Step 2: Define the default operation and setpoint --\nwhen no other operation is being requested."
  # "Step 1: Initialize motors, sersors, and other resources\nof the subsystem outside the loop. Publish the refnums\nfor testing. Wire directly into the loop."
  # "Loop: carries out operation using setpoints, and checks notifier to determine what to do next. Use a timed loop if low timing jitter is key."
  # "Tip: Sometimes it is useful to read sensors and update\ndashboard or globals independent of the control loop."
  n1 = call "Initialize 8 NEO Swerve Drive.vi"() -> ("Motors"=w2:T14)  [unwired: 10 in, 1 out]
  n2 = Unbundle(w2) -> ("Pigeon2"=w1:T21, "Radii (ft)"=w3:T23)  [unwired: 2 out]
  n3 = call "Drive Controller Initialization.vi"("Subsystem Name"=w8, "Default Command"=w4) -> ("Current Command"=w6:T27)  [unwired: 9 in]
  n4 = disable-structure shown="Enabled" {
    disable-tunnel: w3 -> [w10 _]
    disable-tunnel: w2 -> [w9 _]
    frame Disabled {
      n5 = call "Odometry.vi"("Radii (ft)"=w10, "Motors"=w9) -> ()  [unwired: 10 in]
    }
    frame Enabled {
    }
  }
  n6 = vi-ref "Reserve Drive.vi"() -> (w5:refnum<vi>)
  n7 = while {
    shift-right: [w33] -> _
    shift-left: w6 -> [w24]
    tunnel: [w40] -> _
    tunnel: "error in" -> [_]
    tunnel: w5 -> [_]
    tunnel: w2 -> [w31]
    tunnel: w3 -> [w34]
    tunnel: w1 -> [w17]
    i -> [w40]
    stop <- FALSE stop-if-true
    w13 = 0.0 ("element")
    # "Updates metatag2 data for alignment (limelight 4 only)"
    # "Current Command"
    # "Finished? &\nWait Time"
    n8 = Unbundle(w24) -> ("SubSystem Data"=w27:T12, w25:cluster{"Start Time (ms)":u32, "Iterations":i32})  [unwired: 1 out]
    n9 = global write "Robot Global Data.vi" "Drive Controller Data"(w24) -> ()
    n10 = Unbundle By Name(w27) -> ("Operation"=w21:T6, "Robot Velocities"=w35:T13, "Auto Data"=w30:T33, "Left side"=w23:bool, "Angle Align"=w22:bool, "Tag ID"=w18:i32)
    n11 = Tick Count (ms)() -> (millisecond timer value=w26:u32)
    n12 = call "Is Value Changed.vim"("value"=w21) -> ("changed or first call?"=w20:bool)
    n13 = case shown="\"Reef Align\"" w21 {
      selector: w21 -> [w49 _ w77 _ w127 w426]
      tunnel: [w61 -1.0 ("Infinite") 100.0 100.0 ("Infinite") w156 20.0 ("Infinite")] -> w39
      tunnel: [w56 FALSE ("ignore previous (F)") w76 TRUE ("ignore previous (F)") w160 w425] -> w38
      tunnel: w25 -> [w60 _ _ w95 _ _]
      tunnel: w26 -> [w55 _ _ _ _ _]
      tunnel: w35 -> [w53 _ _ _ w157 _]
      tunnel: w31 -> [w51 w67 w84 w93 w159 w428]
      tunnel: w34 -> [_ _ _ _ _ _]
      tunnel: [w54 _ _ _ _ _] -> w32
      tunnel: w27 -> [_ _ _ _ _ _]
      tunnel: w30 -> [_ _ w82 _ _ _]
      tunnel: w23 -> [_ _ _ _ w158 _]
      tunnel: w22 -> [_ _ _ _ w155 _]
      tunnel: w20 -> [w48 _ _ _ _ _]
      tunnel: "Auto PID Constants" -> [_ _ w75 _ w128 w429]
      tunnel: w18 -> [_ _ _ _ w119 _]
      frame "Immediate" {
        w61 = 100.0  # Wait ms
        n14 = Unbundle(w60) -> ("Start Time (ms)"=w59:u32)  [unwired: 1 out]
        n15 = Subtract(x=w55, y=w59) -> (x-y=w58:u32)
        n16 = global read "Robot Global Data.vi" "Drive Conditions"() -> (w52:T34)
        n17 = Greater?(x=w58, y=u32 50) -> (0:w56:bool)
        n18 = call "NEO Swerve Drive.vi"("PID Constants"="Immediate PID Constants", "Configure?"=w48, "Operation"=w49, "Drive Conditions"=w52, "Robot Velocities"=w53, "Swerve Drive"=w51) -> ("Pod Setpoints (ft/s and deg)"=w54:T35)  [unwired: 5 in]
      }
      frame "Reserve", Default {
        # "TODO: remove lmao"
        n19 = Unbundle(w67) -> ("Drive Motors (NEO)"=w66:T15, "Steer Motors (NEO)"=w65:T15)  [unwired: 2 out]
        n20 = disable-structure shown="Disabled" {
          disable-tunnel: w66 -> [w74 _]
          disable-tunnel: w65 -> [w73 _]
          disable-tunnel: FALSE ("Add Angle Offsets?") -> [w72 _]
          disable-tunnel: T11 {"Left Front"=0.0, "Left Back"=0.0, "Right Front"=0.0, "Right Back"=0.0} ("Setpoints") -> [w71 _]
          disable-tunnel: Spark_MAX_Control_Type."Percent VBus" ("Reserve Control Mode") -> [w70 _]
          frame Disabled {
            n21 = call "NEO Set Output.vi"("Control Mode"=w70, "Setpoints"=w71, "Motors"=w74) -> ()  [unwired: 9 in]
            n22 = call "NEO Set Output.vi"("For Steer Motors?"=w72, "Control Mode"=w70, "Setpoints"=w71, "Motors"=w73) -> ()  [unwired: 8 in]
          }
          frame Enabled {
          }
        }
      }
      frame "Auto" {
        n23 = global read "Robot Global Data.vi" "Drive Controller Data"() -> (w81:T27)
        n24 = Unbundle(w81) -> (w80:cluster{"Start Time (ms)":u32, "Iterations":i32})  [unwired: 2 out]
        n25 = Unbundle(w80) -> ("Start Time (ms)"=w79:u32)  [unwired: 1 out]
        n26 = call "Is Value Changed.vim"("value"=w79) -> ("changed or first call?"=w78:bool)
        n27 = case shown="True" w78 {
          tunnel: w82 -> [_ w90]
          tunnel: w84 -> [_ w91]
          tunnel: w77 -> [_ w89]
          tunnel: [FALSE ("Auto Done?") w88] -> w76
          tunnel: w75 -> [_ w87]
          frame False {
            n28 = Wait (ms)(milliseconds to wait=u32 200) -> ()  [unwired: 1 out]
          }
          frame True {
            n29 = call "Auto Play Path.vi"("PID Constants"=w87, "Operation"=w89, "Auto Data"=w90, "Motors"=w91) -> ("Auto Done?"=w88:bool)  [unwired: 7 in]
          }
        }
      }
      frame "Calibrate" {
        n30 = call "Detect Steering Misalignment.vi"("Motors In"=w93) -> ("Motors Out"=w92:T14)  [unwired: 10 in]
        n31 = Unbundle(w95) -> ("Start Time (ms)"=w94:u32)  [unwired: 1 out]
        n32 = while {
          tunnel: w92 -> [w102]
          tunnel: w94 -> [w107]
          stop <- w108 stop-if-true
          n33 = call "ThroughBore Calibration.vi"("Motors"=w102) -> ("error out"=w99:errorcluster, "Steering Angles"=→"(Calibration) Steering Angles":cluster{"LF":dbl, "LB":dbl, "RF":dbl, "RB":dbl})  [unwired: 9 in]
          n34 = Tick Count (ms)() -> (millisecond timer value=w106:u32)
          n35 = Subtract(x=w106, y=w107) -> (x-y=w105:u32)
          n36 = Less?(x=w105, y=u32 3000) -> (x < y?=w103:bool)
          n37 = Unbundle(w99) -> ("code"=w98:i32)  [unwired: 2 out]
          n38 = Or(x=w99, y=w103) -> (x .or. y?=w108:bool)
          n39 = call <vilib>:"WPI_UtilitiesFRC Build Error.vi"("error code"=w98, "chain levels to remove (1)"=0) -> ()  [unwired: 3 in, 11 out]
        }
      }
      frame "Old Reef Align" {
        (unwired) dbl[] [-1.0, -1.0, -1.0, -1.0, -1.0, -60.0, 0.0, 60.0, 120.0, 180.0, 240.0, -1.0, -1.0, -1.0, -1.0, -1.0, 60.0, 0.0, -60.0, -120.0, -180.0, -240.0]
        # "TODO: add in for astra"
        # "x"
        # "y"
        # "th"
        n40 = Quotient & Remainder(x=w119, y=i8 2) -> (x-y*floor(x/y)=w117:i32)  [unwired: 1 out]
        n41 = global read "Robot Global Data.vi" "Robot Mode"() -> (w122:T29)
        n42 = Equal To 0?(x=w117) -> (x = 0?=w116:bool)
        n43 = Equal?(x=w122, y=WPI_DriverStationRobotMode2."Autonomous Enabled") -> (x = y?=w120:bool)
        n44 = Select(t="Even_Tags", s=w116, f="Odd_Tags") -> (s? t:f=w112:string)
        n45 = Select(t=w112, s=w120, f="All_Tags") -> (s? t:f=w110:string)
        n46 = call-poly <vilib>:"NT Write Value.vi"("value"=w110, "name"="limelight-four_PipelineName") -> ("error out"=w109:errorcluster)  [unwired: 9 in]
        n47 = call-poly <vilib>:"NT Read Value.vi"("error in"=w109, "name"="/limelight-astra/botpose_targetspace") -> ("value"=w146:dbl[])  [unwired: 7 in, 2 out]
        n48 = call-poly <vilib>:"NT Read Value.vi"("error in"=w109, "name"="/limelight-four/botpose_targetspace") -> ("value"=w143:dbl[])  [unwired: 7 in, 2 out]
        n49 = call-poly <vilib>:"NT Read Value.vi"("error in"=w109, "name"="/limelight-astra/tid") -> ("value"=w149:dbl)  [unwired: 7 in, 2 out]
        n50 = call-poly <vilib>:"NT Read Value.vi"("error in"=w109, "name"="/limelight-four/tid") -> ("value"=w152:dbl)  [unwired: 7 in, 2 out]
        n51 = Index Array(array=w143, index #1=0 ("index"), index #2=2 ("index"), index #3=4 ("index")) -> (element #1=w134:dbl, element #2=w133:dbl, element #3=w132:dbl)
        n52 = Index Array(array=w146, index #1=0 ("index"), index #2=2 ("index"), index #3=4 ("index")) -> (element #1=w139:dbl, element #2=w138:dbl, element #3=w137:dbl)
        n53 = disable-structure shown="Disabled" {
          disable-tunnel: w139 -> [w162 _]
          disable-tunnel: w134 -> [w161 _]
          frame Disabled {
            n54 = Bundle("Numeric"=w162, "Numeric"=w161) -> (→"Waveform Chart":cluster{"Numeric":dbl, "Numeric":dbl})  [unwired: 1 in]
          }
          frame Enabled {
          }
        }
        n55 = Less Or Equal To 0?(x=w149) -> (x <= 0?=w153:bool)
        n56 = Less Or Equal To 0?(x=w152) -> (x <= 0?=w129:bool)
        n57 = Not And(1:w153, 2:w129) -> (0:w154:bool)
        n58 = Select(t=w152, s=w153, f=w149) -> (s? t:f=w123:dbl)
        n59 = Decrement(x=w123) -> (x-1=w126:dbl)
        n60 = Index Array(array=dbl[] [-1.0, -1.0, -1.0, -1.0, -1.0, -60.0, 0.0, 60.0, 120.0, 180.0, -120.0, -1.0, -1.0, -1.0, -1.0, -1.0, 60.0, 0.0, -60.0, -120.0, -180.0, -240.0] ("Array"), index=w126) -> (element=w124:dbl)
        n61 = disable-structure shown="Disabled" {
          disable-tunnel: [w224 w333] -> w160
          disable-tunnel: w159 -> [w204 w335]
          disable-tunnel: w158 -> [w194 w318]
          disable-tunnel: w157 -> [w193 _]
          disable-tunnel: [w192 _] -> w156
          disable-tunnel: w155 -> [w191 _]
          disable-tunnel: w154 -> [w186 _]
          disable-tunnel: w124 -> [w185 w320]
          disable-tunnel: w153 -> [w184 _]
          disable-tunnel: w152 -> [w183 _]
          disable-tunnel: w146 -> [w182 w363]
          disable-tunnel: w143 -> [w181 w362]
          disable-tunnel: [w178 _] -> w142
          disable-tunnel: w139 -> [_ _]
          disable-tunnel: w138 -> [_ _]
          disable-tunnel: w137 -> [_ _]
          disable-tunnel: w134 -> [w173 _]
          disable-tunnel: w133 -> [w172 _]
          disable-tunnel: w132 -> [w171 _]
          disable-tunnel: "Left X Setpoint" -> [w165 w323]
          disable-tunnel: "Right X Setpoint" -> [w164 w364]
          disable-tunnel: w129 -> [_ w332]
          disable-tunnel: w128 -> [_ w336]
          disable-tunnel: w127 -> [_ w334]
          disable-tunnel: w123 -> [_ w319]
          frame Disabled {
            # "negate removed"
            # "removed negate"
            # "-0.6041666667"
            # "distance from center to limelight"
            # "meters to ft"
            # "0 is left and right, 2 is front and back"
            n62 = Not(x=w184) -> (.not. x?=w174:bool)
            n63 = Select(t=w182, s=w174, f=w181) -> (s? t:f=w187:dbl[])
            n64 = Unbundle By Name(w204) -> ("Pigeon2"=w218:T21)
            n65 = Decrement(x=w183) -> (x-1=w208:dbl)
            n66 = Bundle("Left X Setpoint"=w165, "Left Y Setpoint"="Left Y Setpoint") -> (w197:T36)  [unwired: 1 in]
            n67 = Bundle("Right X Setpoint"=w164, "Right Y Setpoint"="Right Y Setpoint") -> (w195:T37)  [unwired: 1 in]
            n68 = Index Array(array=dbl[] [-1.0, -1.0, -1.0, -1.0, -1.0, -60.0, 0.0, 60.0, 120.0, 180.0, 240.0, -1.0, -1.0, -1.0, -1.0, -1.0, 60.0, 0.0, -60.0, -120.0, -180.0, -240.0], index=w208) -> (element=w207:dbl)
            n69 = call "Generate Trajectory for Alignment.vi"("th"=w172, "y"=w171, "x"=w173) -> ("Trajectory Data Out"=w170:T4)  [unwired: 7 in, 1 out]
            "Trajectory Data Compare" <- w170
            n70 = call-poly <vilib>:"CTRE_Phoenix_Pigeon2_GetStatus.vi"("PigeonIMUDevRef"=w218) -> ("Yaw Pitch Roll"=w219:cluster{"Yaw":dbl, "Pitch":dbl, "Roll":dbl})  [unwired: 8 in, 2 out]
            n71 = Select(t=w197, s=w194, f=w195) -> (s? t:f=w196:T37)
            n72 = Unbundle(w219) -> ("Yaw"=w210:dbl)  [unwired: 2 out]
            n73 = Add(x=180.0, y=w207) -> (x+y=w190:dbl)
            n74 = Subtract(x=w210, y=w190) -> (x-y=w211:dbl)
            n75 = Multiply(x=w187, y=3.28083 ("x")) -> (x*y=w221:dbl[])
            n76 = Unbundle(w196) -> ("Right X Setpoint"=w176:dbl)  [unwired: 1 out]
            n77 = Index Array(array=w170, index=0) -> (element=w168:T38)
            n78 = expression code="(x/180.0)*pi" "degrees to radians"(w211) -> (w217:dbl)
            n79 = Unbundle By Name(w168) -> ("Traj Vel Points"=w167:T39)
            n80 = Index Array(array=w221, index=0) -> (element=w212:dbl)
            n81 = Sine(x=w217) -> (sin(x)=w216:dbl)
            n82 = Not Equal To 0?(x=w212) -> (x != 0?=w213:bool)
            n83 = for {
              tunnel: w167 -> [w226] mode=indexing
              tunnel: [w225] -> w166 mode=indexing
              n84 = Unbundle By Name(w226) -> ("V"=w225:dbl)
            }
            "Trajectory Velocity" <- w166
            n85 = Multiply(x=w216, y=0.168275) -> (x*y=w214:dbl)
            n86 = Add(x=w214, y=w212) -> (x+y=w175:dbl)
            n87 = Select(t=w175, s=w213, f=0.0) -> (s? t:f=w202:dbl)
            n88 = Unbundle By Name("Deadband") -> ("X (ft)"=w203:dbl)
            n89 = call "Align Velocity.vi"("Period"="Period", "Translational Setpoints"=w176, "AprilTag Pos"=w202, "Deadband"=w203, "Velocity Max"="Velocity Max", "Acceleration Max"="Acceleration Max") -> ("At Setpoint?"=w180:bool, "Array size"=w198:i32, "Velocity values"=w177:dbl[])  [unwired: 1 in]
            n90 = Not(x=w180) -> (.not. x?=w179:bool)
            n91 = case shown="True" w186 {
              tunnel: [FALSE w241] -> w224
              tunnel: w177 -> [_ w250]
              tunnel: w179 -> [_ w249]
              tunnel: w204 -> [w231 w242]
              tunnel: "Period" -> [_ w238]
              tunnel: w185 -> [_ w239]
              tunnel: w198 -> [_ w248]
              tunnel: w193 -> [w232 _]
              tunnel: [20.0 -1.0] -> w192
              tunnel: w191 -> [_ w243]
              tunnel: w176 -> [_ w240]
              tunnel: ["nah we cool" "yeah :("] -> w178
              tunnel: w177 -> [_ w236]
              frame False {
                n92 = call "NEO Swerve Drive.vi"("Drive Conditions"=cluster{"Field Centric":bool, "Reef Align":bool} {"Field Centric"=TRUE, "Reef Align"=FALSE}, "Robot Velocities"=w232, "Swerve Drive"=w231) -> ()  [unwired: 8 in, 1 out]
              }
              frame True {
                n93 = call "Trapezoid Align.vi"(4:w243, "Motors"=w242, "Array size"=w248, "Period"=w238, "Go Up?"="Go Up?", 9:w239, "Boolean 3"=w249, "Velocity values"=w250) -> ("Boolean 2"=w246:bool, "Boolean"=w245:bool)  [unwired: 2 in]
                n94 = And(x="PID enabled", y=w246) -> (x .and. y?=w235:bool)
                n95 = case shown="True" w235 {
                  tunnel: [FALSE w257] -> w244
                  tunnel: w243 -> [_ w256]
                  tunnel: w242 -> [_ w255]
                  tunnel: w240 -> [_ w254]
                  tunnel: w238 -> [_ w253]
                  tunnel: w239 -> [_ w252]
                  frame False {
                  }
                  frame True {
                    n96 = node-c288(w253) -> (w259:T30)
                    n97 = timed-loop {
                      timing: w259 -> [_]
                      timing-out: [_] -> w258
                      tunnel: [w298] -> w257
                      tunnel: w256 -> [w289]
                      tunnel: w255 -> [w288]
                      tunnel: w254 -> [w284]
                      tunnel: w252 -> [w266]
                      stop <- w298 stop-if-true
                      w278 = 3.28083 ("x")
                      n98 = node-c288() -> ()  [unwired: 1 in, 1 out]
                      n99 = call-poly <vilib>:"NT Read Value.vi"("name"="/limelight-four/botpose_targetspace") -> ("value"=w263:dbl[])  [unwired: 8 in, 2 out]
                      n100 = call-poly <vilib>:"NT Read Value.vi"("name"="/limelight-four/botpose_targetspace") -> ("value"=w264:dbl[])  [unwired: 8 in, 2 out]
                      n101 = global read "Robot Global Data.vi" "Robot Velocities"() -> (w295:T13)
                      n102 = call-poly <vilib>:"NT Read Value.vi"("name"="/limelight-four/tid") -> ("value"=w282:dbl)  [unwired: 8 in, 2 out]
                      n103 = call-poly <vilib>:"NT Read Value.vi"("name"="/limelight-astra/tid") -> ("value"=w267:dbl)  [unwired: 8 in, 2 out]
                      n104 = Unbundle By Name(w295) -> ("Y Velocity"=w293:dbl)
                      n105 = Equal?(x=w282, y=w266) -> (x = y?=w261:bool)
                      n106 = Equal?(x=w267, y=w266) -> (x = y?=w268:bool)
                      n107 = Select(t=w264, s=w261, f=w263) -> (s? t:f=w262:dbl[])
                      n108 = Index Array(array=w262, index #1=0 ("index"), index #2=2 ("index")) -> (element #1=w285:dbl, element #2=w279:dbl)
                      n109 = Multiply(x=w285, y=w278) -> (x*y=w281:dbl)
                      n110 = Multiply(x=w278, y=w279) -> (x*y=w277:dbl)
                      n111 = Multiply(x=w277, y="Int per ft") -> (x*y=w275:dbl)
                      n112 = Absolute Value(x=w275) -> (abs(x)=w274:dbl)
                      n113 = Round Toward -Infinity(1:w274) -> (0:w273:dbl)
                      n114 = Add(x=w273, y=4.0) -> (x+y=w271:dbl)
                      n115 = call <vilib>:"Median Filter PtByPt.vi"("rank"=w271, "x"=w281) -> ("Filtered x"=w260:dbl)  [unwired: 2 in, 1 out]
                      n116 = Bundle("Filtered x"=w260, "Right X Setpoint"=w284) -> (→"Waveform Chart":T40)  [unwired: 1 in]
                      n117 = Or(x=w261, y=w268) -> (x .or. y?=w269:bool)
                      n118 = case shown="True" w269 {
                        tunnel: [0.0 ("output") w305] -> w286
                        tunnel: w284 -> [_ w304]
                        tunnel: w260 -> [_ w302]
                        frame False {
                        }
                        frame True {
                          n119 = call <vilib>:"Parallel PID (DBL).vi"("output range"=cluster{"high":dbl, "low":dbl} {"high"=10.0, "low"=-10.0}, "PID gains"="PID gains", "process variable"=w302, "setpoint"=w304) -> ("output"=w305:dbl)  [unwired: 4 in, 3 out]
                        }
                      }
                      "PID Out" <- w286
                      n120 = Bundle("output"=w286, "Y Velocity"=w293, 0.0) -> (w292:cluster{"output":dbl, "Y Velocity":dbl, dbl})  [unwired: 1 in]
                      n121 = call "NEO Swerve Drive.vi"(6:w289, "Operation"="Operation", 8:w266, "Drive Conditions"=cluster{"Field Centric":bool, "Reef Align":bool} {"Field Centric"=TRUE, "Reef Align"=TRUE}, "Robot Velocities"=w292, "Swerve Drive"=w288) -> ()  [unwired: 5 in, 1 out]
                      n122 = global read "Robot Global Data.vi" "Aligning?"() -> (w299:bool)
                      n123 = node-c288() -> ()  [unwired: 1 in, 1 out]
                      n124 = Not(x=w299) -> (.not. x?=w298:bool)
                    }
                    n125 = node-c288(w258) -> ()  [unwired: 1 out]
                  }
                }
                n126 = Or(x=w244, y=w245) -> (x .or. y?=w241:bool)
                "Trapezoid Profile" <- w236
              }
            }
          }
          frame Enabled {
            # "TODO: check?"
            # "Limelight 4 can't see?"
            # "TODO:  fix using limelight four only"
            n127 = Select(t=w363, s=w332, f=w362) -> (s? t:f=w361:dbl[])
            n128 = Index Array(array=w361, index #1=0 ("index"), index #2=2 ("index"), index #3=4 ("index")) -> (element #1=w325:dbl, element #2=w329:dbl, element #3=w357:dbl)
            n129 = Multiply(x=w329, y=3.28084) -> (x*y=w328:dbl)
            n130 = disable-structure shown="Enabled" {
              disable-tunnel: w332 -> [w380 w381]
              disable-tunnel: [w377 w382] -> w331
              disable-tunnel: w328 -> [w375 w382]
              disable-tunnel: [_ w381] -> w322
              frame Disabled {
                # "this \"subtraction\" always changes just\nthe y-component, which doesn't account\nfor rotation"
                n131 = Select(t=1.416667 ("x"), s=w380, f=1.166667) -> (s? t:f=w376:dbl)
                n132 = Add(x=w375, y=w376) -> (x+y=w377:dbl)
              }
              frame Enabled {
              }
            }
            n133 = Multiply(x=3.28084 ("y"), y=w325) -> (x*y=w324:dbl)
            n134 = disable-structure shown="Enabled" {
              disable-tunnel: w322 -> [w373 _]
              disable-tunnel: [w370 "Y Setpoint"] -> w321
              frame Disabled {
                n135 = Select(t=-1.416667 ("x"), s=w373, f=-1.166667) -> (s? t:f=w370:dbl)
              }
              frame Enabled {
              }
            }
            n136 = Select(t=w323, s=w318, f=w364) -> (s? t:f=w356:dbl)
            n137 = Bundle("Right X Setpoint"=w356, "Y Setpoint"=w321, 0.0) -> (w354:T41)  [unwired: 1 in]
            n138 = Select(t="Left PID Setpoint", s=w318, f="Right PID Setpoint") -> (s? t:f=w315:dbl)
            n139 = call "Generate Trajectory for Alignment.vi"("Setpoints"=w354, "th"=w357, "y"=w331, "x"=w324) -> ("Trajectory Data Out"=w312:T4)  [unwired: 6 in, 1 out]
            "Trajectory Data Out" <- w312
            n140 = Index Array(array=w312) -> (element=w314:T38)  [unwired: 1 in]
            n141 = Unbundle By Name(w314) -> ("Traj Vel Points"=w367:T39, "Traj Pos Points"=w313:cluster{"x":dbl, "y":dbl, "th":dbl}[])
            n142 = for {
              tunnel: w367 -> [w409] mode=indexing
              tunnel: [w408] -> w366 mode=indexing
              tunnel: [w406] -> w353 mode=indexing
              tunnel: [w407] -> w348 mode=indexing
              tunnel: [w403] -> w350 mode=indexing
              tunnel: [w406] -> w352 mode=indexing
              tunnel: [w405] -> w340 mode=indexing
              n143 = Unbundle By Name(w409) -> ("V vector.x"=w406:dbl, "V vector.y"=w404:dbl, "Omega"=w407:dbl, "V"=w405:dbl)
              n144 = Negate(x=w404) -> (-x=w403:dbl)
              n145 = Bundle("x"=w406, w403, "Omega"=w407) -> (w408:cluster{"x":dbl, dbl, "Omega":dbl})  [unwired: 1 in]
            }
            "Enabled X Velocity" <- w353
            "Enabled Omega" <- w348
            "Enabled Y Velocity" <- w350
            "Enabled VMag" <- w340
            n146 = Add Array Elements(numeric array=w340) -> (sum=w339:dbl)
            n147 = Add Array Elements(numeric array=w350) -> (sum=w349:dbl)
            n148 = Multiply(x=w339, y=0.02) -> (x*y=→"VMag Sum":dbl)
            n149 = Multiply(x=w349, y=0.02) -> (x*y=→"Sum Y":dbl)
            n150 = Add Array Elements(numeric array=w352) -> (sum=w351:dbl)
            n151 = Multiply(x=0.02, y=w351) -> (x*y=→"Sum X":dbl)
            n152 = Bundle By Name(cluster=T33 {"Auto Velocities"=[], "Auto Positions"=[], "Auto Commands"=[], "Zero Velocity?"=[]} ("Auto Data"), "Auto Velocities"=w366, "Auto Positions"=w313) -> (w365:T33)
            n153 = Add Array Elements(numeric array=w348) -> (sum=w345:dbl)
            n154 = Multiply(x=w345, y=0.02) -> (x*y=→"Sum Angle":dbl)
            n155 = disable-structure shown="Enabled" {
              disable-tunnel: enum16{"Start", "Wait"}."Start" ("Synchronization") -> [w384 _]
              disable-tunnel: w365 -> [w383 w391]
              disable-tunnel: w336 -> [_ w393]
              disable-tunnel: w335 -> [_ w392]
              disable-tunnel: w334 -> [_ w390]
              disable-tunnel: [_ w389] -> w333
              disable-tunnel: "Freeze Align?" -> [_ w388]
              disable-tunnel: w320 -> [_ w387]
              disable-tunnel: w319 -> [_ w386]
              disable-tunnel: w315 -> [_ w385]
              frame Disabled {
                n156 = call "Play Path.vi"("Synchronization"=w384, "Auto Data"=w383) -> ()  [unwired: 9 in, 1 out]
              }
              frame Enabled {
                n157 = case shown="False" w388 {
                  tunnel: w393 -> [w401 _]
                  tunnel: w392 -> [w400 _]
                  tunnel: w391 -> [w399 _]
                  tunnel: w390 -> [w398 _]
                  tunnel: [w397 TRUE ("Auto Done?")] -> w389
                  tunnel: w387 -> [w396 _]
                  tunnel: w386 -> [w395 _]
                  tunnel: w385 -> [w394 _]
                  frame False {
                    n158 = call "Reef Align Play Path.vi"("PID setpoint"=w394, "Tag ID"=w395, "PID Constants"=w401, "Operation"=w398, "Auto Data"=w399, "Motors"=w400, "AprilTag Offset"=w396) -> ("Auto Done?"=w397:bool)  [unwired: 4 in]
                  }
                  frame True {
                  }
                }
              }
            }
          }
        }
        "Weird Aligning Code?" <- w142
      }
      frame "Reef Align" {
        # "meters to feet"
        # "ToDo list:\n-test take back half algerithym (spelling hard) to repalce PID on the fly\n-clean controller and other parts\n-import to a new project starting with the templete code to make it easier for season to season use\n-fix visualizer so robot is facing initial direction\n-add in field map to visualizer"
        # "reads in limlight values"
        # "velocity limits (update to desired amount with new robot)"
        # "change to desired end location"
        # "difference in positions"
        # "constants of 0 for naming and ease"
        # "Gathers velocities into auto velocities to run\nflips Y velocity to make robot drive forwards"
        # "1 is X position\n0 is Y position\n5 is theta"
        n159 = call-poly <vilib>:"NT Read Value.vi"("name"="/limelight-four/botpose_wpiblue") -> ("value"=w421:dbl[])  [unwired: 8 in, 2 out]
        n160 = Index Array(array=w421, index #1=1 ("index"), index #2=0 ("index"), index #3=5 ("index")) -> (element #1=w416:dbl, element #2=w415:dbl, element #3=w437:dbl)
        n161 = Bundle("Numeric"=w416, "Numeric"=w415) -> (w420:cluster{"Numeric":dbl, "Numeric":dbl})  [unwired: 1 in]
        n162 = Multiply(x=3.28084, y=w420) -> (x*y=w419:cluster{"Numeric":dbl, "Numeric":dbl})
        n163 = Unbundle(w419) -> ("Numeric"=w418:dbl, "Numeric"=w417:dbl)
        n164 = Bundle(cluster=cluster{"X":dbl, "Y":dbl, "Theta":dbl} {"X"=0.0, "Y"=0.0, "Theta"=0.0}, "X"=w418, "Y"=w417, "Theta"=w437) -> (w410:cluster{"X":dbl, "Y":dbl, "Theta":dbl})
        n165 = call "Field Cord Generate Trajectory for Alignment.vi"("Initial Postion"=w410, "Final Postion"="Final Postion", "Limits"="Limits") -> ("Error"=→"Error":T42, "Trajectory Data Out"=w433:T4)  [unwired: 2 out]
        n166 = Index Array(array=w433) -> (element=w434:T38)  [unwired: 1 in]
        n167 = Unbundle By Name(w434) -> ("Traj Vel Points"=w432:T39, "Traj Pos Points"=w431:cluster{"x":dbl, "y":dbl, "th":dbl}[])
        n168 = for {
          tunnel: [w445] -> w414 mode=indexing
          tunnel: w432 -> [w442] mode=indexing
          n169 = Unbundle By Name(w442) -> ("V vector.x"=w443:dbl, "V vector.y"=w441:dbl, "Omega"=w444:dbl)
          n170 = Bundle("x"=w443, "y"=w441, "Omega"=w444) -> (w445:cluster{"x":dbl, "y":dbl, "Omega":dbl})  [unwired: 1 in]
        }
        n171 = Negate(x=w414) -> (-x=w411:cluster{"x":dbl, "y":dbl, "Omega":dbl}[])
        n172 = Bundle By Name(cluster=T33 {"Auto Velocities"=[], "Auto Positions"=[], "Auto Commands"=[], "Zero Velocity?"=[]} ("Auto Data"), "Auto Velocities"=w411, "Auto Positions"=w431) -> (w427:T33)
        n173 = call "Reef Align Play Path Field Position.vi"("PID Constants swerve"=w429, "Operation"=w426, "Auto Data"=w427, "Motors"=w428) -> ("Align Good?"=w425:bool)
      }
    }
    n174 = call-poly <vilib>:"CTRE_Phoenix_Pigeon2_GetStatus.vi"("PigeonIMUDevRef"=w17) -> ("Yaw Pitch Roll"=w16:cluster{"Yaw":dbl, "Pitch":dbl, "Roll":dbl})  [unwired: 8 in, 2 out]
    n175 = Unbundle By Name(w16) -> ("Yaw"=w11:dbl)
    "Yaw" <- w11
    n176 = Build Array(w11, w13, w13, 15.0 ("element"), w13, w13) -> (w15:dbl[])
    n177 = call-poly <vilib>:"NT Write Value.vi"("value"=w15, "name"="/limelight-four/robot_orientation_set") -> ()  [unwired: 9 in, 1 out]
    n178 = disable-structure shown="Enabled" {
      disable-tunnel: w32 -> [w45 _]
      disable-tunnel: w31 -> [w42 _]
      frame Disabled {
        n179 = call "NEO Get Sensor Values.vi"("Swerve Motors"=w42) -> ("Steer Angles (degrees)"=w43:T11, "Drive Velocities (ft/s)"=w44:T11)  [unwired: 9 in]
        n180 = call "Swerve Drive Visuals.vi"("Steer Angles (degrees)"=w43, "Drive Velocities (ft/s)"=w44, "Pod Setpoints (ft/s and deg)"=w45) -> ("Swerve Visualizer"=→"Swerve Visualizer":cluster{dbl[], dbl[]}[], "Pod Comparisons (Diff -> Setpoint - Actual)"=→"Pod Comparisons (Diff -> Setpoint - Actual)":T10)  [unwired: 7 in]
      }
      frame Enabled {
      }
    }
    n181 = call "Drive Check for New Command.vi"("input cluster"=w24, "Wait time (ms)"=w39, "Finished?"=w38) -> ("Completion"=w29:T25, "Subsystem Name"=w36:string, "Current Command"=w28:T12, "Initial Trace String"=w37:string, "Next Command"=w33:T43)  [unwired: 4 in]
    n182 = case shown="\"Successful\", \"Aborted\"" w29 {
      selector: w29 -> [_ w446]
      tunnel: w37 -> [_ w453]
      tunnel: w28 -> [_ w454]
      tunnel: w36 -> [_ w452]
      frame "Incomplete", Default {
        # "Continuing current command"
      }
      frame "Successful", "Aborted" {
        # "Report and setup for next command"
        n183 = Unbundle By Name(w454) -> ("Robot Velocities.X Velocity"=w450:dbl, "Robot Velocities.Y Velocity"=w451:dbl, "Robot Velocities.Rotational \nVelocity"=w447:dbl)
        n184 = Format Into String(format string="Vx %.1f, Vy %.1f, W %f", initial string=w453, w450, w451, w447) -> (resulting string=w448:string)  [unwired: 1 in, 1 out]
        "Current\nCmd" <- w448
        n185 = call <vilib>:"Trace Results.vi"("Status of previous command"=w446, "Description"=w448, "Subsystem"=w452) -> ()  [unwired: 9 in]
      }
    }
  }
